vi "CUSUM_scan_histogram_20150428.vi"() -> ()   [LabVIEW 2012]
uses:
  <vilib>/Utility/file.llb/Read From Spreadsheet File (DBL).vi
  <vilib>/Analysis/NI_AALPro.lvlib
panel:
  out "Scatter density":i32[][](graph)
  in  "Log t":bool=TRUE
  in  "Min I (pA)":dbl format="%_3g"
  in  "Max I (pA)":dbl=1.0 format="%_3g"
  in  "Current bins":i16=100
  in  "t Min (us)":dbl=1.0 format="%_3g"
  in  "t Max (us)":dbl=2000000.0 format="%_3g"
  in  "t Bins":i16=100
  out "Blockage vs Event time":cluster{"all rows":dbl[], "all rows":dbl[]}(graph)={"all rows"=[1.5563025007672873, 2.041392685158225, 1.9444826721501687, 1.806179973983887, 2.0170333392987803, 1.7323937598229686, 2.1760912590556813, 2.2695129442179165, 2.662757831681574, 2.0644579892269186, 2.1760912590556813, 2.1072099696478683, 1.6434526764861874, 1.380211241711606, 2.2355284469075487, 2.4471580313422194, 1.954242509439325, 1.7481880270062005, 1.9030899869919435, 2.250420002308894, 1.4771212547196624, 2.606381365110605, 2.7781512503836434, 2.1760912590556813, 1.9637878273455553, 3.9774492273823414, 2.0086001717619175, 2.2600713879850747, 2.225309281725863, 2.113943352306837, 3.902655475217926, 1.4771212547196624, 3.45484486000851, 1.7160033436347992, 5.550074181736537, 2.1072099696478683, 2.100370545117563, 2.255272505103306, 2.093421685162235, 1.9242792860618816, 2.6020599913279625, 1.9912260756924949, 1.8325089127062364, 1.7481880270062005, 1.8920946026904804, 2.0, 1.8692317197309762, 1.6434526764861874, 1.9344984512435677, 3.5804687839510017, 2.0170333392987803, 1.792391689498254, 1.9138138523837167, 1.8573324964312685, 3.8290463368531826, 2.3909351071033793, 1.9138138523837167, 2.0569048513364727, 1.9344984512435677, 2.6085260335771943, 3.569373909615046, 2.230448921378274, 1.6812412373755872, 1.5314789170422551, 2.1583624920952498, 1.792391689498254, 1.6232492903979006, 1.9138138523837167, 1.8573324964312685, 1.9344984512435677, 1.7781512503836436, 1.9912260756924949, 1.9030899869919435, 3.1947917577219247, 1.5314789170422551, 1.9444826721501687, 2.230448921378274, 1.5314789170422551, 2.0791812460476247, 1.9822712330395684, 1.9444826721501687, 1.9138138523837167, 1.845098040014257, 1.5563025007672873, 1.9030899869919435, 1.9822712330395684, 2.4885507165004443, 1.6434526764861874, 3.9707187037201894, 1.6020599913279623, 1.7323937598229686, 1.8195439355418688, 1.8920946026904804, 1.6989700043360187, 2.1398790864012365, 2.4471580313422194, 1.414973347970818, 1.662757831681574, 1.9030899869919435, 4.0288151698468875, 4.322260654143684, 1.8692317197309762, 2.1335389083702174, 2.4771212547196626, 1.414973347970818, 3.396548037987132, 1.8325089127062364, 1.9242792860618816, 6.216878141702857], "all rows"=[0.0, 0.466725, 0.526039, 0.471183, 0.48709, 0.480192, 0.48409, 0.485169, 0.497506, 0.568502, 0.497117, 0.506935, 0.466185, 0.30941, 0.262762, 0.516642, 0.578892, 0.481172, 0.221123, 0.478859, 0.568097, 0.261814, 0.458444, 0.504733, 0.43433, 0.563135, 0.581725, 0.386148, 0.494293, 0.379628, 0.439002, 0.509173, 0.287608, 0.718087, 0.344776, 0.470972, 0.513751, 0.523004, 0.445567, 0.528748, 0.51793, 0.563512, 0.490711, 0.421606, 0.377698, 0.503034, 0.462329, 0.428095, 0.323342, 0.48743, 0.602688, 0.457485, 0.37527, 0.476058, 0.431685, 0.5739, 0.53304, 0.570076, 0.465926, 0.497023, 0.567974, 0.579427, 0.493678, 0.355429, 0.336341, 0.486281, 0.334836, 0.577798, 0.602408, 0.423267, 0.54713, 0.322654, 0.511843, 0.365353, 0.548216, 0.278652, 0.437687, 0.455942, 0.307252, 0.48448599999999997, 0.463501, 0.477843, 0.448573, 0.359273, 0.370335, 0.484589, 0.49994, 0.501483, 0.358317, 0.618115, 0.284756, 0.438673, 0.50125, 0.433369, 0.40958, 0.569745, 0.473801, 0.336148, 0.429861, 0.504048, 0.766676, 0.672518, 0.569512, 0.542499, 0.561967, 0.314494, 0.70292, 0.356469, 14.4165]}
  in  "Scatter plot":bool
  in  "stop 2":bool
  in  "stop":bool
  in  "Dwell time min bin":dbl format="%0.2f"
  in  "Dwell time max bin":dbl=20000.0 format="%0.2f"
  in  "Max block min (pA)":dbl format="%0.2f"
  in  "Max block max (pA)":dbl=1.0 format="%0.2f"
  in  "#bins (max block)":i32=50
  out "Max blockage (pA)":T1(graph)={"X Values"=[0.01, 0.03, 0.05, 0.07, 0.09, 0.11, 0.13, 0.15000000000000002, 0.16999999999999998, 0.19, 0.21000000000000002, 0.22999999999999998, 0.25, 0.27, 0.29000000000000004, 0.31, 0.33, 0.35, 0.37, 0.39, 0.41000000000000003, 0.43, 0.45, 0.47, 0.49, 0.51, 0.53, 0.55, 0.5700000000000001, 0.59, 0.61, 0.63, 0.65, 0.67, 0.6900000000000001, 0.71, 0.73, 0.75, 0.77, 0.79, 0.81, 0.8300000000000001, 0.85, 0.87, 0.89, 0.91, 0.93, 0.95, 0.97, 0.99], "Histogram: h(x)"=[0.0, 0.0, 0.0, 0.0, 0.0, 0.0, 0.0, 0.0, 0.0, 0.0, 0.0, 0.0, 0.0, 0.009345794392523364, 0.009345794392523364, 0.0, 0.018691588785046728, 0.018691588785046728, 0.06542056074766354, 0.009345794392523364, 0.056074766355140186, 0.028037383177570093, 0.06542056074766354, 0.07476635514018691, 0.09345794392523364, 0.14018691588785046, 0.14953271028037382, 0.037383177570093455, 0.08411214953271028, 0.06542056074766354, 0.018691588785046728, 0.009345794392523364, 0.0, 0.009345794392523364, 0.018691588785046728, 0.009345794392523364, 0.0, 0.0, 0.009345794392523364, 0.0, 0.0, 0.0, 0.0, 0.0, 0.0, 0.0, 0.0, 0.0, 0.0, 0.0]}
  out "Dwell time (us)":cluster{"Axis":dbl[], dbl[]}[](graph)=[{"Axis"=[200.0, 600.0, 1000.0, 1400.0, 1800.0, 2200.0, 2600.0, 3000.0, 3400.0, 3800.0, 4200.0, 4600.0, 5000.0, 5400.0, 5800.0, 6200.0, 6600.0, 7000.0, 7400.0, 7800.0, 8200.0, 8600.0, 9000.0, 9400.0, 9800.0, 10200.0, 10600.0, 11000.0, 11400.0, 11800.0, 12200.0, 12600.0, 13000.0, 13400.0, 13800.0, 14200.0, 14600.0, 15000.0, 15400.0, 15800.0, 16200.0, 16600.0, 17000.0, 17400.0, 17800.0, 18200.0, 18600.0, 19000.0, 19400.0, 19800.0], [91.0, 5.0, 0.0, 1.0, 0.0, 0.0, 1.0, 1.0, 0.0, 2.0, 0.0, 0.0, 0.0, 0.0, 0.0, 0.0, 1.0, 0.0, 0.0, 1.0, 0.0, 0.0, 0.0, 2.0, 0.0, 0.0, 1.0, 0.0, 0.0, 0.0, 0.0, 0.0, 0.0, 0.0, 0.0, 0.0, 0.0, 0.0, 0.0, 0.0, 0.0, 0.0, 0.0, 0.0, 0.0, 0.0, 0.0, 0.0, 0.0, 0.0]}, {"Axis"=[200.0, 600.0, 1000.0, 1400.0, 1800.0, 2200.0, 2600.0, 3000.0, 3400.0, 3800.0, 4200.0, 4600.0, 5000.0, 5400.0, 5800.0, 6200.0, 6600.0, 7000.0, 7400.0, 7800.0, 8200.0, 8600.0, 9000.0, 9400.0, 9800.0, 10200.0, 10600.0, 11000.0, 11400.0, 11800.0, 12200.0, 12600.0, 13000.0, 13400.0, 13800.0, 14200.0, 14600.0, 15000.0, 15400.0, 15800.0, 16200.0, 16600.0, 17000.0, 17400.0, 17800.0, 18200.0, 18600.0, 19000.0, 19400.0, 19800.0], [0.8584905660377359, 0.04716981132075472, 0.0, 0.009433962264150943, 0.0, 0.0, 0.009433962264150943, 0.009433962264150943, 0.0, 0.018867924528301886, 0.0, 0.0, 0.0, 0.0, 0.0, 0.0, 0.009433962264150943, 0.0, 0.0, 0.009433962264150943, 0.0, 0.0, 0.0, 0.018867924528301886, 0.0, 0.0, 0.009433962264150943, 0.0, 0.0, 0.0, 0.0, 0.0, 0.0, 0.0, 0.0, 0.0, 0.0, 0.0, 0.0, 0.0, 0.0, 0.0, 0.0, 0.0, 0.0, 0.0, 0.0, 0.0, 0.0, 0.0]}]
  out "min dwell time":dbl=24.0
  out "max dwell time":dbl=1647700.0
  in  "#bins (dwell)":i32=50
  in  "Max blockage histogram":bool
  in  "Dwell time histogram":bool
  out "Events analysed":i32
  out "sum (dummy check)":dbl=0.9807673664328832
  out "event length":i32=823856
  out "Histogram":i32[](array[numeric])
  out "Levels histogram":cluster{"Axis":dbl[], dbl[]}(graph)={"Axis"=[-2925.0, -2775.0, -2625.0, -2475.0, -2325.0, -2175.0, -2025.0, -1875.0, -1725.0, -1575.0, -1425.0, -1275.0, -1125.0, -975.0, -825.0, -675.0, -525.0, -375.0, -225.0, -75.0], [0.0, 0.0, 0.0, 0.0, 0.0, 0.0, 0.0, 0.0, 0.0, 0.0, 0.0, 0.00022756755787289165, 0.6987230927229675, 0.000277542494399701, 0.001647841378534532, 0.026337860039121676, 0.1949290617247068, 0.049781111930785465, 0.008843288584494536, 0.0]}
  out "Cumulative histogram":i32[](array[numeric])
  in  "# bins":i32=20
  in  "Min current (pA)":dbl=-3000.0 format="%0.2f"
  in  "Max current (pA)":dbl format="%0.2f"
  in  "CUSUM levels histogram":bool
  out "Event details":dbl[](array[numeric])=[12.97, 40.0, 729.134, 1.0] caption="Time (s)\n      Length (us)\nMax block (pA)   \n           # levels"
  out "CUSUM event":path=path "D:/Analysis/CUSUM_github/CUSUM/output/events/event_00000.csv"
  out "CUSUM event":cluster{"Y":dbl[], "Y":dbl[]}[](graph)=[{"Y"=[0.0, 2.0, 4.0, 6.0, 8.0, 10.0, 12.0, 14.0, 16.0, 18.0, 20.0, 22.0, 24.0, 26.0, 28.0, 30.0, 32.0, 34.0, 36.0, 38.0, 40.0, 42.0, 44.0, 46.0, 48.0, 50.0, 52.0, 54.0, 56.0, 58.0, 60.0, 62.0, 64.0, 66.0, 68.0, 70.0, 72.0, 74.0, 76.0, 78.0, 80.0, 82.0, 84.0, 86.0, 88.0, 90.0, 92.0, 94.0, 96.0, 98.0, 100.0, 102.0, 104.0, 106.0, 108.0, 110.0, 112.0, 114.0, 116.0, 118.0, 120.0, 122.0, 124.0, 126.0, 128.0, 130.0, 132.0, 134.0, 136.0, 138.0, 140.0, 142.0, 144.0, 146.0, 148.0, 150.0, 152.0, 154.0, 156.0, 158.0, 160.0, 162.0, 164.0, 166.0, 168.0, 170.0, 172.0, 174.0, 176.0, 178.0, 180.0, 182.0, 184.0, 186.0, 188.0, 190.0, 192.0, 194.0, 196.0, 198.0, 200.0, 202.0, 204.0, 206.0, 208.0, 210.0, 212.0, 214.0, 216.0, 218.0, 220.0, 222.0, 224.0, 226.0, 228.0, 230.0, 232.0, 234.0, 236.0, 238.0, 240.0, 242.0, 244.0, 246.0, 248.0, 250.0, 252.0, 254.0, 256.0, 258.0, 260.0, 262.0, 264.0, 266.0, 268.0, 270.0, 272.0, 274.0, 276.0, 278.0, 280.0, 282.0, 284.0, 286.0, 288.0, 290.0, 292.0, 294.0, 296.0, 298.0, 300.0, 302.0, 304.0, 306.0, 308.0, 310.0, 312.0, 314.0, 316.0, 318.0, 320.0, 322.0, 324.0, 326.0, 328.0, 330.0, 332.0, 334.0, 336.0, 338.0, 340.0, 342.0, 344.0, 346.0, 348.0, 350.0, 352.0, 354.0, 356.0, 358.0, 360.0, 362.0, 364.0, 366.0, 368.0, 370.0, 372.0, 374.0, 376.0, 378.0, 380.0, 382.0, 384.0, 386.0, 388.0, 390.0, 392.0, 394.0, 396.0, 398.0, 400.0, 402.0, 404.0, 406.0, 408.0, 410.0, 412.0, 414.0, 416.0, 418.0, 420.0, 422.0, 424.0, 426.0, 428.0, 430.0, 432.0, 434.0, 436.0, 438.0], "Y"=[-1508.27, -1508.27, -1508.27, -1508.27, -1508.27, -1508.27, -1508.27, -1508.27, -1508.27, -1508.27, -1508.27, -1508.27, -1508.27, -1508.27, -1508.27, -1508.27, -1508.27, -1508.27, -1508.27, -1508.27, -1508.27, -1508.27, -1508.27, -1508.27, -1508.27, -1508.27, -1508.27, -1508.27, -1508.27, -1508.27, -1508.27, -1508.27, -1508.27, -1508.27, -1508.27, -1508.27, -1508.27, -1508.27, -1508.27, -1508.27, -1508.27, -1508.27, -1508.27, -1508.27, -1508.27, -1508.27, -1508.27, -1508.27, -1508.27, -1508.27, -1508.27, -1508.27, -1508.27, -1508.27, -1508.27, -1508.27, -1508.27, -1508.27, -1508.27, -1508.27, -1508.27, -1508.27, -1508.27, -1508.27, -1508.27, -1508.27, -1508.27, -1508.27, -1508.27, -1508.27, -1508.27, -1508.27, -1508.27, -1508.27, -1508.27, -1508.27, -1508.27, -1508.27, -1508.27, -1508.27, -1508.27, -1508.27, -1508.27, -1508.27, -1508.27, -1508.27, -1508.27, -1508.27, -1508.27, -1508.27, -1508.27, -1508.27, -1508.27, -1508.27, -1508.27, -1508.27, -772.071, -772.071, -772.071, -772.071, -772.071, -772.071, -772.071, -772.071, -772.071, -772.071, -772.071, -772.071, -772.071, -772.071, -772.071, -772.071, -772.071, -772.071, -772.071, -772.071, -1508.61, -1508.61, -1508.61, -1508.61, -1508.61, -1508.61, -1508.61, -1508.61, -1508.61, -1508.61, -1508.61, -1508.61, -1508.61, -1508.61, -1508.61, -1508.61, -1508.61, -1508.61, -1508.61, -1508.61, -1508.61, -1508.61, -1508.61, -1508.61, -1508.61, -1508.61, -1508.61, -1508.61, -1508.61, -1508.61, -1508.61, -1508.61, -1508.61, -1508.61, -1508.61, -1508.61, -1508.61, -1508.61, -1508.61, -1508.61, -1508.61, -1508.61, -1508.61, -1508.61, -1508.61, -1508.61, -1508.61, -1508.61, -1508.61, -1508.61, -1508.61, -1508.61, -1508.61, -1508.61, -1508.61, -1508.61, -1508.61, -1508.61, -1508.61, -1508.61, -1508.61, -1508.61, -1508.61, -1508.61, -1508.61, -1508.61, -1508.61, -1508.61, -1508.61, -1508.61, -1508.61, -1508.61, -1508.61, -1508.61, -1508.61, -1508.61, -1508.61, -1508.61, -1508.61, -1508.61, -1508.61, -1508.61, -1508.61, -1508.61, -1508.61, -1508.61, -1508.61, -1508.61, -1508.61, -1508.61, -1508.61, -1508.61, -1508.61, -1508.61, -1508.61, -1508.61, -1508.61, -1508.61, -1508.61, -1508.61, -1508.61, -1508.61, -1508.61, -1508.61]}, {"Y"=[0.0, 2.0, 4.0, 6.0, 8.0, 10.0, 12.0, 14.0, 16.0, 18.0, 20.0, 22.0, 24.0, 26.0, 28.0, 30.0, 32.0, 34.0, 36.0, 38.0, 40.0, 42.0, 44.0, 46.0, 48.0, 50.0, 52.0, 54.0, 56.0, 58.0, 60.0, 62.0, 64.0, 66.0, 68.0, 70.0, 72.0, 74.0, 76.0, 78.0, 80.0, 82.0, 84.0, 86.0, 88.0, 90.0, 92.0, 94.0, 96.0, 98.0, 100.0, 102.0, 104.0, 106.0, 108.0, 110.0, 112.0, 114.0, 116.0, 118.0, 120.0, 122.0, 124.0, 126.0, 128.0, 130.0, 132.0, 134.0, 136.0, 138.0, 140.0, 142.0, 144.0, 146.0, 148.0, 150.0, 152.0, 154.0, 156.0, 158.0, 160.0, 162.0, 164.0, 166.0, 168.0, 170.0, 172.0, 174.0, 176.0, 178.0, 180.0, 182.0, 184.0, 186.0, 188.0, 190.0, 192.0, 194.0, 196.0, 198.0, 200.0, 202.0, 204.0, 206.0, 208.0, 210.0, 212.0, 214.0, 216.0, 218.0, 220.0, 222.0, 224.0, 226.0, 228.0, 230.0, 232.0, 234.0, 236.0, 238.0, 240.0, 242.0, 244.0, 246.0, 248.0, 250.0, 252.0, 254.0, 256.0, 258.0, 260.0, 262.0, 264.0, 266.0, 268.0, 270.0, 272.0, 274.0, 276.0, 278.0, 280.0, 282.0, 284.0, 286.0, 288.0, 290.0, 292.0, 294.0, 296.0, 298.0, 300.0, 302.0, 304.0, 306.0, 308.0, 310.0, 312.0, 314.0, 316.0, 318.0, 320.0, 322.0, 324.0, 326.0, 328.0, 330.0, 332.0, 334.0, 336.0, 338.0, 340.0, 342.0, 344.0, 346.0, 348.0, 350.0, 352.0, 354.0, 356.0, 358.0, 360.0, 362.0, 364.0, 366.0, 368.0, 370.0, 372.0, 374.0, 376.0, 378.0, 380.0, 382.0, 384.0, 386.0, 388.0, 390.0, 392.0, 394.0, 396.0, 398.0, 400.0, 402.0, 404.0, 406.0, 408.0, 410.0, 412.0, 414.0, 416.0, 418.0, 420.0, 422.0, 424.0, 426.0, 428.0, 430.0, 432.0, 434.0, 436.0, 438.0], "Y"=[-1591.0, -1421.0, -1377.0, -1507.0, -1587.0, -1555.0, -1525.0, -1599.0, -1675.0, -1611.0, -1522.0, -1485.0, -1503.0, -1599.0, -1521.0, -1314.0, -1273.0, -1460.0, -1603.0, -1536.0, -1415.0, -1464.0, -1619.0, -1713.0, -1672.0, -1504.0, -1475.0, -1558.0, -1529.0, -1446.0, -1411.0, -1400.0, -1501.0, -1613.0, -1571.0, -1472.0, -1484.0, -1538.0, -1437.0, -1313.0, -1363.0, -1463.0, -1461.0, -1390.0, -1323.0, -1322.0, -1513.0, -1657.0, -1618.0, -1466.0, -1355.0, -1465.0, -1560.0, -1517.0, -1441.0, -1459.0, -1398.0, -1396.0, -1455.0, -1489.0, -1574.0, -1630.0, -1561.0, -1525.0, -1483.0, -1555.0, -1600.0, -1542.0, -1463.0, -1484.0, -1550.0, -1559.0, -1489.0, -1380.0, -1454.0, -1640.0, -1731.0, -1722.0, -1512.0, -1454.0, -1525.0, -1579.0, -1514.0, -1447.0, -1563.0, -1594.0, -1434.0, -1364.0, -1457.0, -1674.0, -1679.0, -1552.0, -1467.0, -1450.0, -1532.0, -1533.0, -1326.0, -1135.0, -1060.0, -1000.0, -855.0, -654.0, -599.0, -706.0, -794.0, -828.0, -804.0, -746.0, -802.0, -892.0, -790.0, -635.0, -657.0, -792.0, -907.0, -857.0, -924.0, -1202.0, -1410.0, -1325.0, -1275.0, -1315.0, -1432.0, -1525.0, -1512.0, -1491.0, -1390.0, -1342.0, -1478.0, -1581.0, -1497.0, -1437.0, -1585.0, -1622.0, -1547.0, -1561.0, -1547.0, -1516.0, -1443.0, -1399.0, -1358.0, -1423.0, -1571.0, -1589.0, -1513.0, -1480.0, -1594.0, -1705.0, -1670.0, -1530.0, -1461.0, -1530.0, -1554.0, -1438.0, -1399.0, -1421.0, -1506.0, -1549.0, -1498.0, -1375.0, -1339.0, -1460.0, -1545.0, -1444.0, -1327.0, -1458.0, -1582.0, -1587.0, -1582.0, -1545.0, -1614.0, -1637.0, -1503.0, -1391.0, -1356.0, -1405.0, -1457.0, -1506.0, -1503.0, -1450.0, -1527.0, -1602.0, -1546.0, -1399.0, -1443.0, -1593.0, -1650.0, -1594.0, -1517.0, -1546.0, -1696.0, -1683.0, -1579.0, -1548.0, -1611.0, -1620.0, -1542.0, -1484.0, -1450.0, -1508.0, -1537.0, -1490.0, -1448.0, -1432.0, -1527.0, -1578.0, -1494.0, -1408.0, -1424.0, -1537.0, -1626.0, -1617.0, -1508.0, -1456.0, -1497.0, -1514.0, -1427.0, -1400.0, -1502.0, -1599.0]}]
  in  "Event Index":i32
  out "All Files in Dir":path[](array[path])=[path "D:/Analysis/CUSUM_github/CUSUM/output/events/event_00000.csv", path "D:/Analysis/CUSUM_github/CUSUM/output/events/event_00001.csv", path "D:/Analysis/CUSUM_github/CUSUM/output/events/event_00004.csv", path "D:/Analysis/CUSUM_github/CUSUM/output/events/event_00009.csv", path "D:/Analysis/CUSUM_github/CUSUM/output/events/event_00011.csv", path "D:/Analysis/CUSUM_github/CUSUM/output/events/event_00013.csv", path "D:/Analysis/CUSUM_github/CUSUM/output/events/event_00015.csv", path "D:/Analysis/CUSUM_github/CUSUM/output/events/event_00016.csv", path "D:/Analysis/CUSUM_github/CUSUM/output/events/event_00018.csv", path "D:/Analysis/CUSUM_github/CUSUM/output/events/event_00019.csv", path "D:/Analysis/CUSUM_github/CUSUM/output/events/event_00020.csv", path "D:/Analysis/CUSUM_github/CUSUM/output/events/event_00022.csv", path "D:/Analysis/CUSUM_github/CUSUM/output/events/event_00024.csv", path "D:/Analysis/CUSUM_github/CUSUM/output/events/event_00025.csv", path "D:/Analysis/CUSUM_github/CUSUM/output/events/event_00027.csv", path "D:/Analysis/CUSUM_github/CUSUM/output/events/event_00031.csv", path "D:/Analysis/CUSUM_github/CUSUM/output/events/event_00032.csv", path "D:/Analysis/CUSUM_github/CUSUM/output/events/event_00034.csv", path "D:/Analysis/CUSUM_github/CUSUM/output/events/event_00035.csv", path "D:/Analysis/CUSUM_github/CUSUM/output/events/event_00038.csv", path "D:/Analysis/CUSUM_github/CUSUM/output/events/event_00041.csv", path "D:/Analysis/CUSUM_github/CUSUM/output/events/event_00043.csv", path "D:/Analysis/CUSUM_github/CUSUM/output/events/event_00044.csv", path "D:/Analysis/CUSUM_github/CUSUM/output/events/event_00046.csv", path "D:/Analysis/CUSUM_github/CUSUM/output/events/event_00047.csv", path "D:/Analysis/CUSUM_github/CUSUM/output/events/event_00048.csv", path "D:/Analysis/CUSUM_github/CUSUM/output/events/event_00049.csv", path "D:/Analysis/CUSUM_github/CUSUM/output/events/event_00051.csv", path "D:/Analysis/CUSUM_github/CUSUM/output/events/event_00053.csv", path "D:/Analysis/CUSUM_github/CUSUM/output/events/event_00054.csv", path "D:/Analysis/CUSUM_github/CUSUM/output/events/event_00056.csv", path "D:/Analysis/CUSUM_github/CUSUM/output/events/event_00057.csv", path "D:/Analysis/CUSUM_github/CUSUM/output/events/event_00060.csv", path "D:/Analysis/CUSUM_github/CUSUM/output/events/event_00061.csv", path "D:/Analysis/CUSUM_github/CUSUM/output/events/event_00062.csv", path "D:/Analysis/CUSUM_github/CUSUM/output/events/event_00063.csv", path "D:/Analysis/CUSUM_github/CUSUM/output/events/event_00068.csv", path "D:/Analysis/CUSUM_github/CUSUM/output/events/event_00069.csv", path "D:/Analysis/CUSUM_github/CUSUM/output/events/event_00070.csv", path "D:/Analysis/CUSUM_github/CUSUM/output/events/event_00072.csv", path "D:/Analysis/CUSUM_github/CUSUM/output/events/event_00074.csv", path "D:/Analysis/CUSUM_github/CUSUM/output/events/event_00076.csv", path "D:/Analysis/CUSUM_github/CUSUM/output/events/event_00077.csv", path "D:/Analysis/CUSUM_github/CUSUM/output/events/event_00078.csv", path "D:/Analysis/CUSUM_github/CUSUM/output/events/event_00079.csv", path "D:/Analysis/CUSUM_github/CUSUM/output/events/event_00080.csv", path "D:/Analysis/CUSUM_github/CUSUM/output/events/event_00081.csv", path "D:/Analysis/CUSUM_github/CUSUM/output/events/event_00082.csv", path "D:/Analysis/CUSUM_github/CUSUM/output/events/event_00084.csv", path "D:/Analysis/CUSUM_github/CUSUM/output/events/event_00087.csv", path "D:/Analysis/CUSUM_github/CUSUM/output/events/event_00089.csv", path "D:/Analysis/CUSUM_github/CUSUM/output/events/event_00093.csv", path "D:/Analysis/CUSUM_github/CUSUM/output/events/event_00094.csv", path "D:/Analysis/CUSUM_github/CUSUM/output/events/event_00096.csv", path "D:/Analysis/CUSUM_github/CUSUM/output/events/event_00098.csv", path "D:/Analysis/CUSUM_github/CUSUM/output/events/event_00101.csv", path "D:/Analysis/CUSUM_github/CUSUM/output/events/event_00102.csv", path "D:/Analysis/CUSUM_github/CUSUM/output/events/event_00103.csv", path "D:/Analysis/CUSUM_github/CUSUM/output/events/event_00108.csv", path "D:/Analysis/CUSUM_github/CUSUM/output/events/event_00109.csv", path "D:/Analysis/CUSUM_github/CUSUM/output/events/event_00111.csv", path "D:/Analysis/CUSUM_github/CUSUM/output/events/event_00114.csv", path "D:/Analysis/CUSUM_github/CUSUM/output/events/event_00120.csv", path "D:/Analysis/CUSUM_github/CUSUM/output/events/event_00121.csv", path "D:/Analysis/CUSUM_github/CUSUM/output/events/event_00122.csv", path "D:/Analysis/CUSUM_github/CUSUM/output/events/event_00128.csv", path "D:/Analysis/CUSUM_github/CUSUM/output/events/event_00130.csv", path "D:/Analysis/CUSUM_github/CUSUM/output/events/event_00131.csv", path "D:/Analysis/CUSUM_github/CUSUM/output/events/event_00132.csv", path "D:/Analysis/CUSUM_github/CUSUM/output/events/event_00133.csv", path "D:/Analysis/CUSUM_github/CUSUM/output/events/event_00134.csv", path "D:/Analysis/CUSUM_github/CUSUM/output/events/event_00137.csv", path "D:/Analysis/CUSUM_github/CUSUM/output/events/event_00138.csv", path "D:/Analysis/CUSUM_github/CUSUM/output/events/event_00139.csv", path "D:/Analysis/CUSUM_github/CUSUM/output/events/event_00142.csv", path "D:/Analysis/CUSUM_github/CUSUM/output/events/event_00143.csv", path "D:/Analysis/CUSUM_github/CUSUM/output/events/event_00146.csv", path "D:/Analysis/CUSUM_github/CUSUM/output/events/event_00148.csv", path "D:/Analysis/CUSUM_github/CUSUM/output/events/event_00152.csv", path "D:/Analysis/CUSUM_github/CUSUM/output/events/event_00155.csv", path "D:/Analysis/CUSUM_github/CUSUM/output/events/event_00156.csv", path "D:/Analysis/CUSUM_github/CUSUM/output/events/event_00164.csv", path "D:/Analysis/CUSUM_github/CUSUM/output/events/event_00166.csv", path "D:/Analysis/CUSUM_github/CUSUM/output/events/event_00167.csv", path "D:/Analysis/CUSUM_github/CUSUM/output/events/event_00171.csv", path "D:/Analysis/CUSUM_github/CUSUM/output/events/event_00172.csv", path "D:/Analysis/CUSUM_github/CUSUM/output/events/event_00176.csv", path "D:/Analysis/CUSUM_github/CUSUM/output/events/event_00177.csv", path "D:/Analysis/CUSUM_github/CUSUM/output/events/event_00178.csv", path "D:/Analysis/CUSUM_github/CUSUM/output/events/event_00181.csv", path "D:/Analysis/CUSUM_github/CUSUM/output/events/event_00187.csv", path "D:/Analysis/CUSUM_github/CUSUM/output/events/event_00189.csv", path "D:/Analysis/CUSUM_github/CUSUM/output/events/event_00193.csv", path "D:/Analysis/CUSUM_github/CUSUM/output/events/event_00195.csv", path "D:/Analysis/CUSUM_github/CUSUM/output/events/event_00196.csv", path "D:/Analysis/CUSUM_github/CUSUM/output/events/event_00197.csv", path "D:/Analysis/CUSUM_github/CUSUM/output/events/event_00203.csv", path "D:/Analysis/CUSUM_github/CUSUM/output/events/event_00204.csv", path "D:/Analysis/CUSUM_github/CUSUM/output/events/event_00205.csv", path "D:/Analysis/CUSUM_github/CUSUM/output/events/event_00208.csv", path "D:/Analysis/CUSUM_github/CUSUM/output/events/event_00209.csv", path "D:/Analysis/CUSUM_github/CUSUM/output/events/event_00210.csv", path "D:/Analysis/CUSUM_github/CUSUM/output/events/event_00211.csv", path "D:/Analysis/CUSUM_github/CUSUM/output/events/event_00212.csv", path "D:/Analysis/CUSUM_github/CUSUM/output/events/event_00213.csv", path "D:/Analysis/CUSUM_github/CUSUM/output/events/event_00216.csv", path "D:/Analysis/CUSUM_github/CUSUM/output/events/event_00218.csv", path "D:/Analysis/CUSUM_github/CUSUM/output/events/event_00221.csv", path "D:/Analysis/CUSUM_github/CUSUM/output/events/event_00222.csv", path "D:/Analysis/CUSUM_github/CUSUM/output/events/event_00223.csv", path "D:/Analysis/CUSUM_github/CUSUM/output/events/event_00230.csv", path "D:/Analysis/CUSUM_github/CUSUM/output/events/event_00232.csv", path "D:/Analysis/CUSUM_github/CUSUM/output/events/event_00233.csv", path "D:/Analysis/CUSUM_github/CUSUM/output/events/event_00234.csv", path "D:/Analysis/CUSUM_github/CUSUM/output/events/event_00238.csv", path "D:/Analysis/CUSUM_github/CUSUM/output/events/event_00240.csv", path "D:/Analysis/CUSUM_github/CUSUM/output/events/event_00247.csv", path "D:/Analysis/CUSUM_github/CUSUM/output/events/event_00249.csv", path "D:/Analysis/CUSUM_github/CUSUM/output/events/event_00255.csv", path "D:/Analysis/CUSUM_github/CUSUM/output/events/event_00257.csv", path "D:/Analysis/CUSUM_github/CUSUM/output/events/event_00258.csv", path "D:/Analysis/CUSUM_github/CUSUM/output/events/event_00264.csv", path "D:/Analysis/CUSUM_github/CUSUM/output/events/event_00265.csv", path "D:/Analysis/CUSUM_github/CUSUM/output/events/event_00267.csv", path "D:/Analysis/CUSUM_github/CUSUM/output/events/event_00268.csv", path "D:/Analysis/CUSUM_github/CUSUM/output/events/event_00271.csv", path "D:/Analysis/CUSUM_github/CUSUM/output/events/event_00273.csv", path "D:/Analysis/CUSUM_github/CUSUM/output/events/event_00280.csv", path "D:/Analysis/CUSUM_github/CUSUM/output/events/event_00285.csv", path "D:/Analysis/CUSUM_github/CUSUM/output/events/event_00286.csv", path "D:/Analysis/CUSUM_github/CUSUM/output/events/event_00287.csv", path "D:/Analysis/CUSUM_github/CUSUM/output/events/event_00288.csv", path "D:/Analysis/CUSUM_github/CUSUM/output/events/event_00289.csv", path "D:/Analysis/CUSUM_github/CUSUM/output/events/event_00290.csv", path "D:/Analysis/CUSUM_github/CUSUM/output/events/event_00291.csv", path "D:/Analysis/CUSUM_github/CUSUM/output/events/event_00294.csv", path "D:/Analysis/CUSUM_github/CUSUM/output/events/event_00297.csv", path "D:/Analysis/CUSUM_github/CUSUM/output/events/event_00300.csv", path "D:/Analysis/CUSUM_github/CUSUM/output/events/event_00302.csv", path "D:/Analysis/CUSUM_github/CUSUM/output/events/event_00305.csv", path "D:/Analysis/CUSUM_github/CUSUM/output/events/event_00306.csv", path "D:/Analysis/CUSUM_github/CUSUM/output/events/event_00307.csv", path "D:/Analysis/CUSUM_github/CUSUM/output/events/event_00308.csv", path "D:/Analysis/CUSUM_github/CUSUM/output/events/event_00310.csv", path "D:/Analysis/CUSUM_github/CUSUM/output/events/event_00313.csv", path "D:/Analysis/CUSUM_github/CUSUM/output/events/event_00317.csv", path "D:/Analysis/CUSUM_github/CUSUM/output/events/event_00319.csv", path "D:/Analysis/CUSUM_github/CUSUM/output/events/event_00322.csv", path "D:/Analysis/CUSUM_github/CUSUM/output/events/event_00323.csv", path "D:/Analysis/CUSUM_github/CUSUM/output/events/event_00324.csv", path "D:/Analysis/CUSUM_github/CUSUM/output/events/event_00325.csv", path "D:/Analysis/CUSUM_github/CUSUM/output/events/event_00328.csv", path "D:/Analysis/CUSUM_github/CUSUM/output/events/event_00331.csv", path "D:/Analysis/CUSUM_github/CUSUM/output/events/event_00332.csv", path "D:/Analysis/CUSUM_github/CUSUM/output/events/event_00333.csv", path "D:/Analysis/CUSUM_github/CUSUM/output/events/event_00335.csv", path "D:/Analysis/CUSUM_github/CUSUM/output/events/event_00336.csv", path "D:/Analysis/CUSUM_github/CUSUM/output/events/event_00337.csv", path "D:/Analysis/CUSUM_github/CUSUM/output/events/event_00339.csv", path "D:/Analysis/CUSUM_github/CUSUM/output/events/event_00344.csv", path "D:/Analysis/CUSUM_github/CUSUM/output/events/event_00345.csv", path "D:/Analysis/CUSUM_github/CUSUM/output/events/event_00351.csv", path "D:/Analysis/CUSUM_github/CUSUM/output/events/event_00352.csv", path "D:/Analysis/CUSUM_github/CUSUM/output/events/event_00354.csv", path "D:/Analysis/CUSUM_github/CUSUM/output/events/event_00355.csv", path "D:/Analysis/CUSUM_github/CUSUM/output/events/event_00356.csv", path "D:/Analysis/CUSUM_github/CUSUM/output/events/event_00361.csv", path "D:/Analysis/CUSUM_github/CUSUM/output/events/event_00362.csv", path "D:/Analysis/CUSUM_github/CUSUM/output/events/event_00365.csv", path "D:/Analysis/CUSUM_github/CUSUM/output/events/event_00367.csv", path "D:/Analysis/CUSUM_github/CUSUM/output/events/event_00369.csv", path "D:/Analysis/CUSUM_github/CUSUM/output/events/event_00373.csv", path "D:/Analysis/CUSUM_github/CUSUM/output/events/event_00374.csv", path "D:/Analysis/CUSUM_github/CUSUM/output/events/event_00376.csv", path "D:/Analysis/CUSUM_github/CUSUM/output/events/event_00377.csv", path "D:/Analysis/CUSUM_github/CUSUM/output/events/event_00378.csv", path "D:/Analysis/CUSUM_github/CUSUM/output/events/event_00380.csv", path "D:/Analysis/CUSUM_github/CUSUM/output/events/event_00381.csv", path "D:/Analysis/CUSUM_github/CUSUM/output/events/event_00387.csv", path "D:/Analysis/CUSUM_github/CUSUM/output/events/event_00388.csv", path "D:/Analysis/CUSUM_github/CUSUM/output/events/event_00389.csv", path "D:/Analysis/CUSUM_github/CUSUM/output/events/event_00390.csv", path "D:/Analysis/CUSUM_github/CUSUM/output/events/event_00391.csv", path "D:/Analysis/CUSUM_github/CUSUM/output/events/event_00397.csv", path "D:/Analysis/CUSUM_github/CUSUM/output/events/event_00398.csv", path "D:/Analysis/CUSUM_github/CUSUM/output/events/event_00399.csv", path "D:/Analysis/CUSUM_github/CUSUM/output/events/event_00400.csv", path "D:/Analysis/CUSUM_github/CUSUM/output/events/event_00402.csv", path "D:/Analysis/CUSUM_github/CUSUM/output/events/event_00403.csv", path "D:/Analysis/CUSUM_github/CUSUM/output/events/event_00404.csv", path "D:/Analysis/CUSUM_github/CUSUM/output/events/event_00409.csv", path "D:/Analysis/CUSUM_github/CUSUM/output/events/event_00410.csv", path "D:/Analysis/CUSUM_github/CUSUM/output/events/event_00414.csv", path "D:/Analysis/CUSUM_github/CUSUM/output/events/event_00417.csv", path "D:/Analysis/CUSUM_github/CUSUM/output/events/event_00418.csv", path "D:/Analysis/CUSUM_github/CUSUM/output/events/event_00421.csv", path "D:/Analysis/CUSUM_github/CUSUM/output/events/event_00425.csv", path "D:/Analysis/CUSUM_github/CUSUM/output/events/event_00426.csv", path "D:/Analysis/CUSUM_github/CUSUM/output/events/event_00432.csv", path "D:/Analysis/CUSUM_github/CUSUM/output/events/event_00433.csv", path "D:/Analysis/CUSUM_github/CUSUM/output/events/event_00434.csv", path "D:/Analysis/CUSUM_github/CUSUM/output/events/event_00436.csv", path "D:/Analysis/CUSUM_github/CUSUM/output/events/event_00437.csv", path "D:/Analysis/CUSUM_github/CUSUM/output/events/event_00440.csv", path "D:/Analysis/CUSUM_github/CUSUM/output/events/event_00441.csv", path "D:/Analysis/CUSUM_github/CUSUM/output/events/event_00447.csv", path "D:/Analysis/CUSUM_github/CUSUM/output/events/event_00452.csv", path "D:/Analysis/CUSUM_github/CUSUM/output/events/event_00455.csv", path "D:/Analysis/CUSUM_github/CUSUM/output/events/event_00460.csv", path "D:/Analysis/CUSUM_github/CUSUM/output/events/event_00461.csv", path "D:/Analysis/CUSUM_github/CUSUM/output/events/event_00464.csv", path "D:/Analysis/CUSUM_github/CUSUM/output/events/event_00466.csv", path "D:/Analysis/CUSUM_github/CUSUM/output/events/event_00467.csv", path "D:/Analysis/CUSUM_github/CUSUM/output/events/event_00469.csv", path "D:/Analysis/CUSUM_github/CUSUM/output/events/event_00471.csv", path "D:/Analysis/CUSUM_github/CUSUM/output/events/event_00472.csv", path "D:/Analysis/CUSUM_github/CUSUM/output/events/event_00473.csv", path "D:/Analysis/CUSUM_github/CUSUM/output/events/event_00474.csv", path "D:/Analysis/CUSUM_github/CUSUM/output/events/event_00476.csv", path "D:/Analysis/CUSUM_github/CUSUM/output/events/event_00477.csv", path "D:/Analysis/CUSUM_github/CUSUM/output/events/event_00478.csv", path "D:/Analysis/CUSUM_github/CUSUM/output/events/event_00480.csv", path "D:/Analysis/CUSUM_github/CUSUM/output/events/event_00484.csv", path "D:/Analysis/CUSUM_github/CUSUM/output/events/event_00485.csv", path "D:/Analysis/CUSUM_github/CUSUM/output/events/event_00487.csv", path "D:/Analysis/CUSUM_github/CUSUM/output/events/event_00488.csv", path "D:/Analysis/CUSUM_github/CUSUM/output/events/event_00490.csv", path "D:/Analysis/CUSUM_github/CUSUM/output/events/event_00495.csv", path "D:/Analysis/CUSUM_github/CUSUM/output/events/event_00501.csv", path "D:/Analysis/CUSUM_github/CUSUM/output/events/event_00504.csv", path "D:/Analysis/CUSUM_github/CUSUM/output/events/event_00506.csv", path "D:/Analysis/CUSUM_github/CUSUM/output/events/event_00507.csv", path "D:/Analysis/CUSUM_github/CUSUM/output/events/event_00508.csv", path "D:/Analysis/CUSUM_github/CUSUM/output/events/event_00509.csv", path "D:/Analysis/CUSUM_github/CUSUM/output/events/event_00510.csv", path "D:/Analysis/CUSUM_github/CUSUM/output/events/event_00512.csv", path "D:/Analysis/CUSUM_github/CUSUM/output/events/event_00515.csv", path "D:/Analysis/CUSUM_github/CUSUM/output/events/event_00516.csv", path "D:/Analysis/CUSUM_github/CUSUM/output/events/event_00517.csv", path "D:/Analysis/CUSUM_github/CUSUM/output/events/event_00525.csv", path "D:/Analysis/CUSUM_github/CUSUM/output/events/event_00526.csv", path "D:/Analysis/CUSUM_github/CUSUM/output/events/event_00527.csv", path "D:/Analysis/CUSUM_github/CUSUM/output/events/event_00531.csv", path "D:/Analysis/CUSUM_github/CUSUM/output/events/event_00533.csv", path "D:/Analysis/CUSUM_github/CUSUM/output/events/event_00534.csv", path "D:/Analysis/CUSUM_github/CUSUM/output/events/event_00535.csv", path "D:/Analysis/CUSUM_github/CUSUM/output/events/event_00539.csv", path "D:/Analysis/CUSUM_github/CUSUM/output/events/event_00540.csv", path "D:/Analysis/CUSUM_github/CUSUM/output/events/event_00544.csv", path "D:/Analysis/CUSUM_github/CUSUM/output/events/event_00547.csv", path "D:/Analysis/CUSUM_github/CUSUM/output/events/event_00548.csv", path "D:/Analysis/CUSUM_github/CUSUM/output/events/event_00551.csv", path "D:/Analysis/CUSUM_github/CUSUM/output/events/event_00553.csv", path "D:/Analysis/CUSUM_github/CUSUM/output/events/event_00556.csv", path "D:/Analysis/CUSUM_github/CUSUM/output/events/event_00557.csv", path "D:/Analysis/CUSUM_github/CUSUM/output/events/event_00558.csv", path "D:/Analysis/CUSUM_github/CUSUM/output/events/event_00561.csv", path "D:/Analysis/CUSUM_github/CUSUM/output/events/event_00563.csv", path "D:/Analysis/CUSUM_github/CUSUM/output/events/event_00564.csv", path "D:/Analysis/CUSUM_github/CUSUM/output/events/event_00566.csv", path "D:/Analysis/CUSUM_github/CUSUM/output/events/event_00567.csv", path "D:/Analysis/CUSUM_github/CUSUM/output/events/event_00568.csv", path "D:/Analysis/CUSUM_github/CUSUM/output/events/event_00569.csv", path "D:/Analysis/CUSUM_github/CUSUM/output/events/event_00570.csv", path "D:/Analysis/CUSUM_github/CUSUM/output/events/event_00576.csv", path "D:/Analysis/CUSUM_github/CUSUM/output/events/event_00577.csv", path "D:/Analysis/CUSUM_github/CUSUM/output/events/event_00580.csv", path "D:/Analysis/CUSUM_github/CUSUM/output/events/event_00585.csv", path "D:/Analysis/CUSUM_github/CUSUM/output/events/event_00586.csv", path "D:/Analysis/CUSUM_github/CUSUM/output/events/event_00589.csv", path "D:/Analysis/CUSUM_github/CUSUM/output/events/event_00592.csv", path "D:/Analysis/CUSUM_github/CUSUM/output/events/event_00595.csv", path "D:/Analysis/CUSUM_github/CUSUM/output/events/event_00597.csv", path "D:/Analysis/CUSUM_github/CUSUM/output/events/event_00598.csv", path "D:/Analysis/CUSUM_github/CUSUM/output/events/event_00599.csv", path "D:/Analysis/CUSUM_github/CUSUM/output/events/event_00606.csv", path "D:/Analysis/CUSUM_github/CUSUM/output/events/event_00608.csv", path "D:/Analysis/CUSUM_github/CUSUM/output/events/event_00609.csv", path "D:/Analysis/CUSUM_github/CUSUM/output/events/event_00610.csv", path "D:/Analysis/CUSUM_github/CUSUM/output/events/event_00611.csv", path "D:/Analysis/CUSUM_github/CUSUM/output/events/event_00614.csv", path "D:/Analysis/CUSUM_github/CUSUM/output/events/event_00615.csv", path "D:/Analysis/CUSUM_github/CUSUM/output/events/event_00616.csv", path "D:/Analysis/CUSUM_github/CUSUM/output/events/event_00617.csv", path "D:/Analysis/CUSUM_github/CUSUM/output/events/event_00618.csv", path "D:/Analysis/CUSUM_github/CUSUM/output/events/event_00624.csv", path "D:/Analysis/CUSUM_github/CUSUM/output/events/event_00625.csv", path "D:/Analysis/CUSUM_github/CUSUM/output/events/event_00626.csv", path "D:/Analysis/CUSUM_github/CUSUM/output/events/event_00628.csv", path "D:/Analysis/CUSUM_github/CUSUM/output/events/event_00630.csv", path "D:/Analysis/CUSUM_github/CUSUM/output/events/event_00632.csv", path "D:/Analysis/CUSUM_github/CUSUM/output/events/event_00633.csv", path "D:/Analysis/CUSUM_github/CUSUM/output/events/event_00634.csv", path "D:/Analysis/CUSUM_github/CUSUM/output/events/event_00635.csv", path "D:/Analysis/CUSUM_github/CUSUM/output/events/event_00636.csv", path "D:/Analysis/CUSUM_github/CUSUM/output/events/event_00638.csv", path "D:/Analysis/CUSUM_github/CUSUM/output/events/event_00640.csv", path "D:/Analysis/CUSUM_github/CUSUM/output/events/event_00649.csv", path "D:/Analysis/CUSUM_github/CUSUM/output/events/event_00655.csv", path "D:/Analysis/CUSUM_github/CUSUM/output/events/event_00659.csv", path "D:/Analysis/CUSUM_github/CUSUM/output/events/event_00666.csv", path "D:/Analysis/CUSUM_github/CUSUM/output/events/event_00669.csv", path "D:/Analysis/CUSUM_github/CUSUM/output/events/event_00670.csv", path "D:/Analysis/CUSUM_github/CUSUM/output/events/event_00673.csv", path "D:/Analysis/CUSUM_github/CUSUM/output/events/event_00679.csv", path "D:/Analysis/CUSUM_github/CUSUM/output/events/event_00694.csv", path "D:/Analysis/CUSUM_github/CUSUM/output/events/event_00698.csv", path "D:/Analysis/CUSUM_github/CUSUM/output/events/event_00700.csv", path "D:/Analysis/CUSUM_github/CUSUM/output/events/event_00701.csv", path "D:/Analysis/CUSUM_github/CUSUM/output/events/event_00702.csv", path "D:/Analysis/CUSUM_github/CUSUM/output/events/event_00703.csv", path "D:/Analysis/CUSUM_github/CUSUM/output/events/event_00707.csv", path "D:/Analysis/CUSUM_github/CUSUM/output/events/event_00708.csv", path "D:/Analysis/CUSUM_github/CUSUM/output/events/event_00709.csv", path "D:/Analysis/CUSUM_github/CUSUM/output/events/event_00710.csv", path "D:/Analysis/CUSUM_github/CUSUM/output/events/event_00713.csv", path "D:/Analysis/CUSUM_github/CUSUM/output/events/event_00716.csv", path "D:/Analysis/CUSUM_github/CUSUM/output/events/event_00717.csv", path "D:/Analysis/CUSUM_github/CUSUM/output/events/event_00718.csv", path "D:/Analysis/CUSUM_github/CUSUM/output/events/event_00720.csv", path "D:/Analysis/CUSUM_github/CUSUM/output/events/event_00721.csv", path "D:/Analysis/CUSUM_github/CUSUM/output/events/event_00723.csv", path "D:/Analysis/CUSUM_github/CUSUM/output/events/event_00724.csv", path "D:/Analysis/CUSUM_github/CUSUM/output/events/event_00726.csv", path "D:/Analysis/CUSUM_github/CUSUM/output/events/event_00728.csv", path "D:/Analysis/CUSUM_github/CUSUM/output/events/event_00731.csv", path "D:/Analysis/CUSUM_github/CUSUM/output/events/event_00732.csv", path "D:/Analysis/CUSUM_github/CUSUM/output/events/event_00733.csv", path "D:/Analysis/CUSUM_github/CUSUM/output/events/event_00735.csv", path "D:/Analysis/CUSUM_github/CUSUM/output/events/event_00736.csv", path "D:/Analysis/CUSUM_github/CUSUM/output/events/event_00739.csv", path "D:/Analysis/CUSUM_github/CUSUM/output/events/event_00740.csv", path "D:/Analysis/CUSUM_github/CUSUM/output/events/event_00746.csv", path "D:/Analysis/CUSUM_github/CUSUM/output/events/event_00747.csv", path "D:/Analysis/CUSUM_github/CUSUM/output/events/event_00749.csv", path "D:/Analysis/CUSUM_github/CUSUM/output/events/event_00750.csv", path "D:/Analysis/CUSUM_github/CUSUM/output/events/event_00751.csv", path "D:/Analysis/CUSUM_github/CUSUM/output/events/event_00752.csv", path "D:/Analysis/CUSUM_github/CUSUM/output/events/event_00753.csv", path "D:/Analysis/CUSUM_github/CUSUM/output/events/event_00754.csv", path "D:/Analysis/CUSUM_github/CUSUM/output/events/event_00755.csv", path "D:/Analysis/CUSUM_github/CUSUM/output/events/event_00760.csv", path "D:/Analysis/CUSUM_github/CUSUM/output/events/event_00761.csv", path "D:/Analysis/CUSUM_github/CUSUM/output/events/event_00762.csv", path "D:/Analysis/CUSUM_github/CUSUM/output/events/event_00763.csv", path "D:/Analysis/CUSUM_github/CUSUM/output/events/event_00764.csv", path "D:/Analysis/CUSUM_github/CUSUM/output/events/event_00765.csv", path "D:/Analysis/CUSUM_github/CUSUM/output/events/event_00766.csv", path "D:/Analysis/CUSUM_github/CUSUM/output/events/event_00767.csv", path "D:/Analysis/CUSUM_github/CUSUM/output/events/event_00768.csv", path "D:/Analysis/CUSUM_github/CUSUM/output/events/event_00769.csv", path "D:/Analysis/CUSUM_github/CUSUM/output/events/event_00770.csv", path "D:/Analysis/CUSUM_github/CUSUM/output/events/event_00771.csv", path "D:/Analysis/CUSUM_github/CUSUM/output/events/event_00772.csv", path "D:/Analysis/CUSUM_github/CUSUM/output/events/event_00774.csv", path "D:/Analysis/CUSUM_github/CUSUM/output/events/event_00778.csv", path "D:/Analysis/CUSUM_github/CUSUM/output/events/event_00779.csv", path "D:/Analysis/CUSUM_github/CUSUM/output/events/event_00780.csv", path "D:/Analysis/CUSUM_github/CUSUM/output/events/event_00790.csv", path "D:/Analysis/CUSUM_github/CUSUM/output/events/event_00795.csv", path "D:/Analysis/CUSUM_github/CUSUM/output/events/event_00801.csv", path "D:/Analysis/CUSUM_github/CUSUM/output/events/event_00803.csv", path "D:/Analysis/CUSUM_github/CUSUM/output/events/event_00804.csv", path "D:/Analysis/CUSUM_github/CUSUM/output/events/event_00815.csv", path "D:/Analysis/CUSUM_github/CUSUM/output/events/event_00816.csv", path "D:/Analysis/CUSUM_github/CUSUM/output/events/event_00819.csv", path "D:/Analysis/CUSUM_github/CUSUM/output/events/event_00823.csv", path "D:/Analysis/CUSUM_github/CUSUM/output/events/event_00824.csv", path "D:/Analysis/CUSUM_github/CUSUM/output/events/event_00833.csv", path "D:/Analysis/CUSUM_github/CUSUM/output/events/event_00835.csv", path "D:/Analysis/CUSUM_github/CUSUM/output/events/event_00836.csv", path "D:/Analysis/CUSUM_github/CUSUM/output/events/event_00837.csv", path "D:/Analysis/CUSUM_github/CUSUM/output/events/event_00839.csv", path "D:/Analysis/CUSUM_github/CUSUM/output/events/event_00842.csv", path "D:/Analysis/CUSUM_github/CUSUM/output/events/event_00844.csv", path "D:/Analysis/CUSUM_github/CUSUM/output/events/event_00845.csv", path "D:/Analysis/CUSUM_github/CUSUM/output/events/event_00847.csv", path "D:/Analysis/CUSUM_github/CUSUM/output/events/event_00849.csv", path "D:/Analysis/CUSUM_github/CUSUM/output/events/event_00850.csv", path "D:/Analysis/CUSUM_github/CUSUM/output/events/event_00853.csv", path "D:/Analysis/CUSUM_github/CUSUM/output/events/event_00856.csv", path "D:/Analysis/CUSUM_github/CUSUM/output/events/event_00857.csv", path "D:/Analysis/CUSUM_github/CUSUM/output/events/event_00858.csv", path "D:/Analysis/CUSUM_github/CUSUM/output/events/event_00859.csv", path "D:/Analysis/CUSUM_github/CUSUM/output/events/event_00860.csv", path "D:/Analysis/CUSUM_github/CUSUM/output/events/event_00861.csv", path "D:/Analysis/CUSUM_github/CUSUM/output/events/event_00864.csv", path "D:/Analysis/CUSUM_github/CUSUM/output/events/event_00865.csv", path "D:/Analysis/CUSUM_github/CUSUM/output/events/event_00866.csv", path "D:/Analysis/CUSUM_github/CUSUM/output/events/event_00867.csv", path "D:/Analysis/CUSUM_github/CUSUM/output/events/event_00875.csv", path "D:/Analysis/CUSUM_github/CUSUM/output/events/event_00877.csv", path "D:/Analysis/CUSUM_github/CUSUM/output/events/event_00878.csv", path "D:/Analysis/CUSUM_github/CUSUM/output/events/event_00879.csv", path "D:/Analysis/CUSUM_github/CUSUM/output/events/event_00882.csv", path "D:/Analysis/CUSUM_github/CUSUM/output/events/event_00884.csv", path "D:/Analysis/CUSUM_github/CUSUM/output/events/event_00885.csv", path "D:/Analysis/CUSUM_github/CUSUM/output/events/event_00886.csv", path "D:/Analysis/CUSUM_github/CUSUM/output/events/event_00887.csv", path "D:/Analysis/CUSUM_github/CUSUM/output/events/event_00888.csv", path "D:/Analysis/CUSUM_github/CUSUM/output/events/event_00890.csv", path "D:/Analysis/CUSUM_github/CUSUM/output/events/event_00894.csv", path "D:/Analysis/CUSUM_github/CUSUM/output/events/event_00898.csv", path "D:/Analysis/CUSUM_github/CUSUM/output/events/event_00900.csv", path "D:/Analysis/CUSUM_github/CUSUM/output/events/event_00903.csv", path "D:/Analysis/CUSUM_github/CUSUM/output/events/event_00905.csv", path "D:/Analysis/CUSUM_github/CUSUM/output/events/event_00906.csv", path "D:/Analysis/CUSUM_github/CUSUM/output/events/event_00907.csv", path "D:/Analysis/CUSUM_github/CUSUM/output/events/event_00908.csv", path "D:/Analysis/CUSUM_github/CUSUM/output/events/event_00909.csv", path "D:/Analysis/CUSUM_github/CUSUM/output/events/event_00913.csv", path "D:/Analysis/CUSUM_github/CUSUM/output/events/event_00915.csv", path "D:/Analysis/CUSUM_github/CUSUM/output/events/event_00916.csv", path "D:/Analysis/CUSUM_github/CUSUM/output/events/event_00920.csv", path "D:/Analysis/CUSUM_github/CUSUM/output/events/event_00921.csv", path "D:/Analysis/CUSUM_github/CUSUM/output/events/event_00924.csv", path "D:/Analysis/CUSUM_github/CUSUM/output/events/event_00925.csv", path "D:/Analysis/CUSUM_github/CUSUM/output/events/event_00930.csv", path "D:/Analysis/CUSUM_github/CUSUM/output/events/event_00934.csv", path "D:/Analysis/CUSUM_github/CUSUM/output/events/event_00938.csv", path "D:/Analysis/CUSUM_github/CUSUM/output/events/event_00939.csv", path "D:/Analysis/CUSUM_github/CUSUM/output/events/event_00941.csv", path "D:/Analysis/CUSUM_github/CUSUM/output/events/event_00942.csv", path "D:/Analysis/CUSUM_github/CUSUM/output/events/event_00946.csv", path "D:/Analysis/CUSUM_github/CUSUM/output/events/event_00949.csv", path "D:/Analysis/CUSUM_github/CUSUM/output/events/event_00950.csv", path "D:/Analysis/CUSUM_github/CUSUM/output/events/event_00951.csv", path "D:/Analysis/CUSUM_github/CUSUM/output/events/event_00953.csv", path "D:/Analysis/CUSUM_github/CUSUM/output/events/event_00960.csv", path "D:/Analysis/CUSUM_github/CUSUM/output/events/event_00962.csv", path "D:/Analysis/CUSUM_github/CUSUM/output/events/event_00966.csv", path "D:/Analysis/CUSUM_github/CUSUM/output/events/event_00969.csv", path "D:/Analysis/CUSUM_github/CUSUM/output/events/event_00973.csv", path "D:/Analysis/CUSUM_github/CUSUM/output/events/event_00977.csv", path "D:/Analysis/CUSUM_github/CUSUM/output/events/event_00980.csv", path "D:/Analysis/CUSUM_github/CUSUM/output/events/event_00981.csv", path "D:/Analysis/CUSUM_github/CUSUM/output/events/event_00982.csv", path "D:/Analysis/CUSUM_github/CUSUM/output/events/event_00986.csv", path "D:/Analysis/CUSUM_github/CUSUM/output/events/event_00988.csv", path "D:/Analysis/CUSUM_github/CUSUM/output/events/event_00993.csv", path "D:/Analysis/CUSUM_github/CUSUM/output/events/event_00995.csv", path "D:/Analysis/CUSUM_github/CUSUM/output/events/event_00997.csv", path "D:/Analysis/CUSUM_github/CUSUM/output/events/event_00999.csv", path "D:/Analysis/CUSUM_github/CUSUM/output/events/event_01003.csv", path "D:/Analysis/CUSUM_github/CUSUM/output/events/event_01005.csv", path "D:/Analysis/CUSUM_github/CUSUM/output/events/event_01007.csv", path "D:/Analysis/CUSUM_github/CUSUM/output/events/event_01009.csv", path "D:/Analysis/CUSUM_github/CUSUM/output/events/event_01015.csv", path "D:/Analysis/CUSUM_github/CUSUM/output/events/event_01020.csv", path "D:/Analysis/CUSUM_github/CUSUM/output/events/event_01021.csv", path "D:/Analysis/CUSUM_github/CUSUM/output/events/event_01023.csv", path "D:/Analysis/CUSUM_github/CUSUM/output/events/event_01028.csv", path "D:/Analysis/CUSUM_github/CUSUM/output/events/event_01032.csv", path "D:/Analysis/CUSUM_github/CUSUM/output/events/event_01034.csv", path "D:/Analysis/CUSUM_github/CUSUM/output/events/event_01036.csv", path "D:/Analysis/CUSUM_github/CUSUM/output/events/event_01037.csv", path "D:/Analysis/CUSUM_github/CUSUM/output/events/event_01038.csv", path "D:/Analysis/CUSUM_github/CUSUM/output/events/event_01042.csv", path "D:/Analysis/CUSUM_github/CUSUM/output/events/event_01044.csv", path "D:/Analysis/CUSUM_github/CUSUM/output/events/event_01045.csv", path "D:/Analysis/CUSUM_github/CUSUM/output/events/event_01046.csv", path "D:/Analysis/CUSUM_github/CUSUM/output/events/event_01047.csv", path "D:/Analysis/CUSUM_github/CUSUM/output/events/event_01048.csv", path "D:/Analysis/CUSUM_github/CUSUM/output/events/event_01049.csv", path "D:/Analysis/CUSUM_github/CUSUM/output/events/event_01054.csv", path "D:/Analysis/CUSUM_github/CUSUM/output/events/event_01057.csv", path "D:/Analysis/CUSUM_github/CUSUM/output/events/event_01062.csv", path "D:/Analysis/CUSUM_github/CUSUM/output/events/event_01064.csv", path "D:/Analysis/CUSUM_github/CUSUM/output/events/event_01066.csv", path "D:/Analysis/CUSUM_github/CUSUM/output/events/event_01068.csv", path "D:/Analysis/CUSUM_github/CUSUM/output/events/event_01071.csv", path "D:/Analysis/CUSUM_github/CUSUM/output/events/event_01076.csv", path "D:/Analysis/CUSUM_github/CUSUM/output/events/event_01081.csv", path "D:/Analysis/CUSUM_github/CUSUM/output/events/event_01083.csv", path "D:/Analysis/CUSUM_github/CUSUM/output/events/event_01084.csv", path "D:/Analysis/CUSUM_github/CUSUM/output/events/event_01086.csv", path "D:/Analysis/CUSUM_github/CUSUM/output/events/event_01093.csv", path "D:/Analysis/CUSUM_github/CUSUM/output/events/event_01094.csv", path "D:/Analysis/CUSUM_github/CUSUM/output/events/event_01096.csv", path "D:/Analysis/CUSUM_github/CUSUM/output/events/event_01097.csv", path "D:/Analysis/CUSUM_github/CUSUM/output/events/event_01099.csv", path "D:/Analysis/CUSUM_github/CUSUM/output/events/event_01101.csv", path "D:/Analysis/CUSUM_github/CUSUM/output/events/event_01102.csv", path "D:/Analysis/CUSUM_github/CUSUM/output/events/event_01108.csv"]
  out "Total # of events":i32=484
  in  "CUSUM event summary file":path=path "D:/Analysis/CUSUM_github/CUSUM/output/events.csv"
  # "'Page up/down' to \nscan through events"
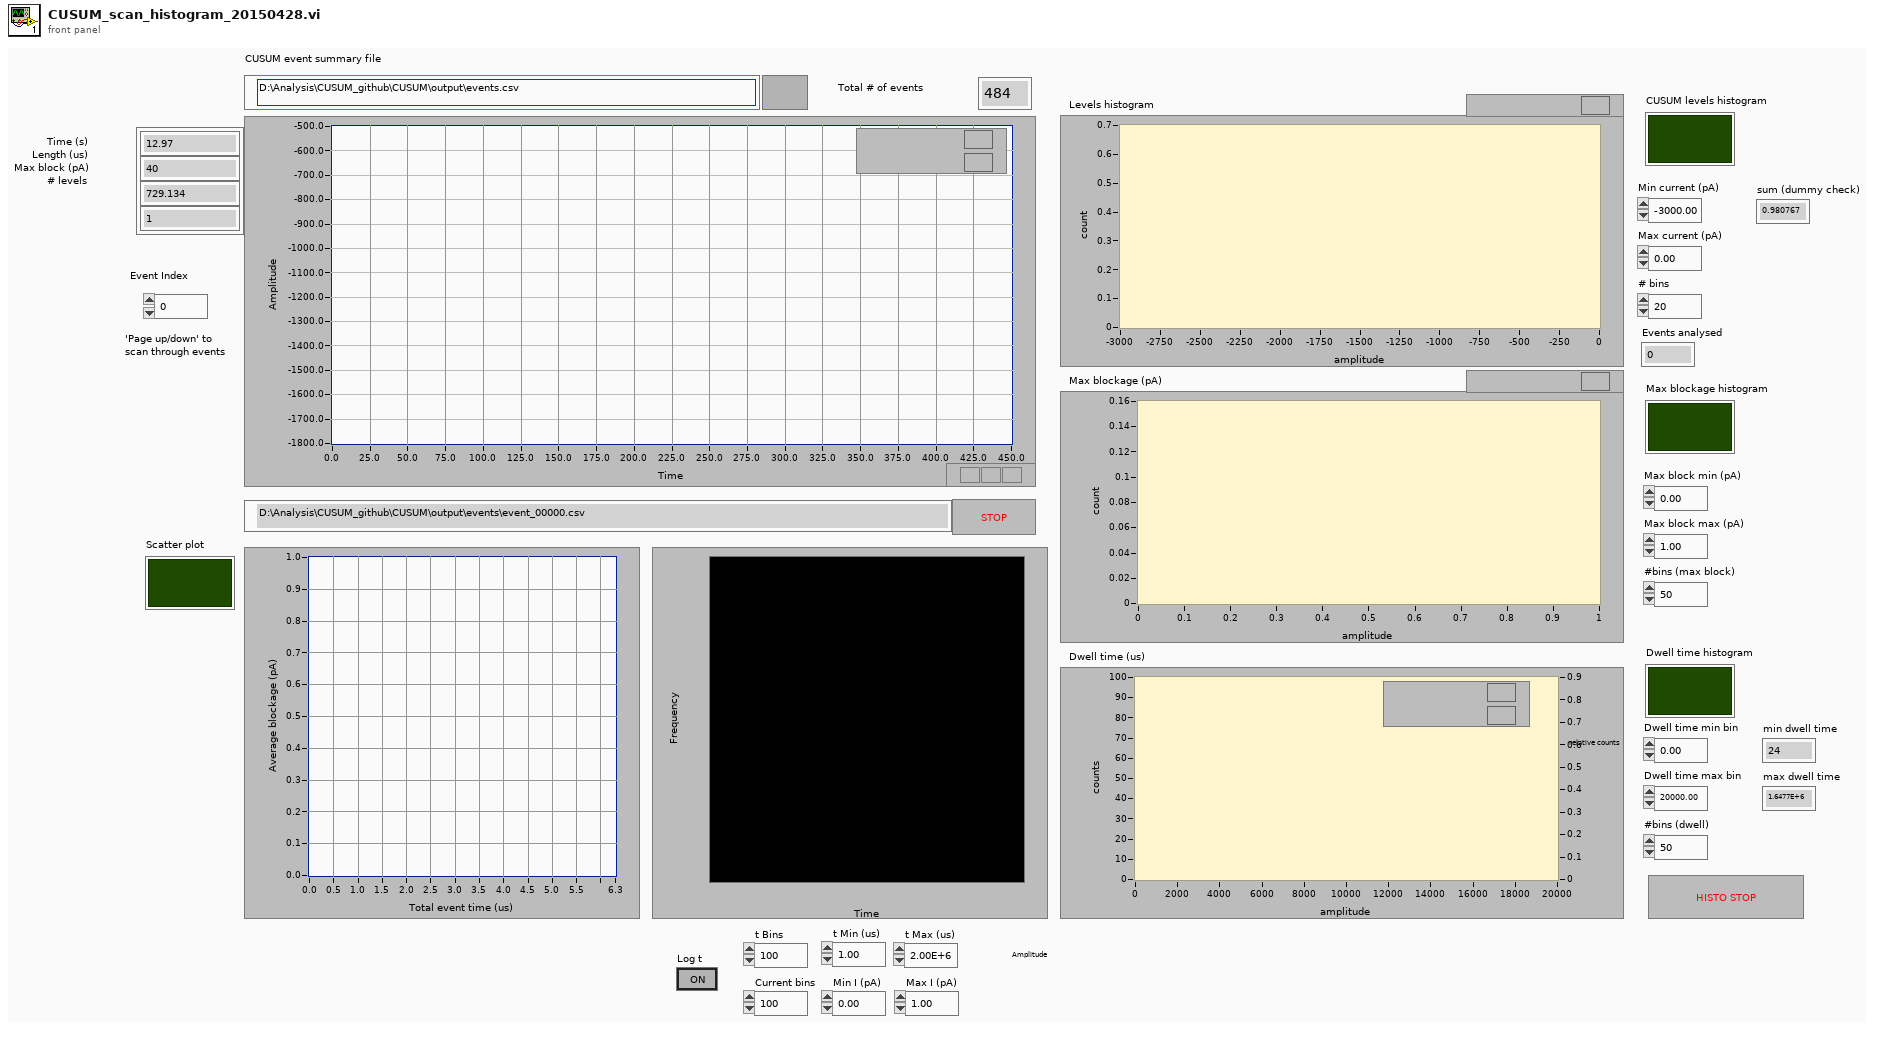
[diagram p1: front panel]
types:
  T1 = cluster{"X Values":dbl[], "Histogram: h(x)":dbl[]}
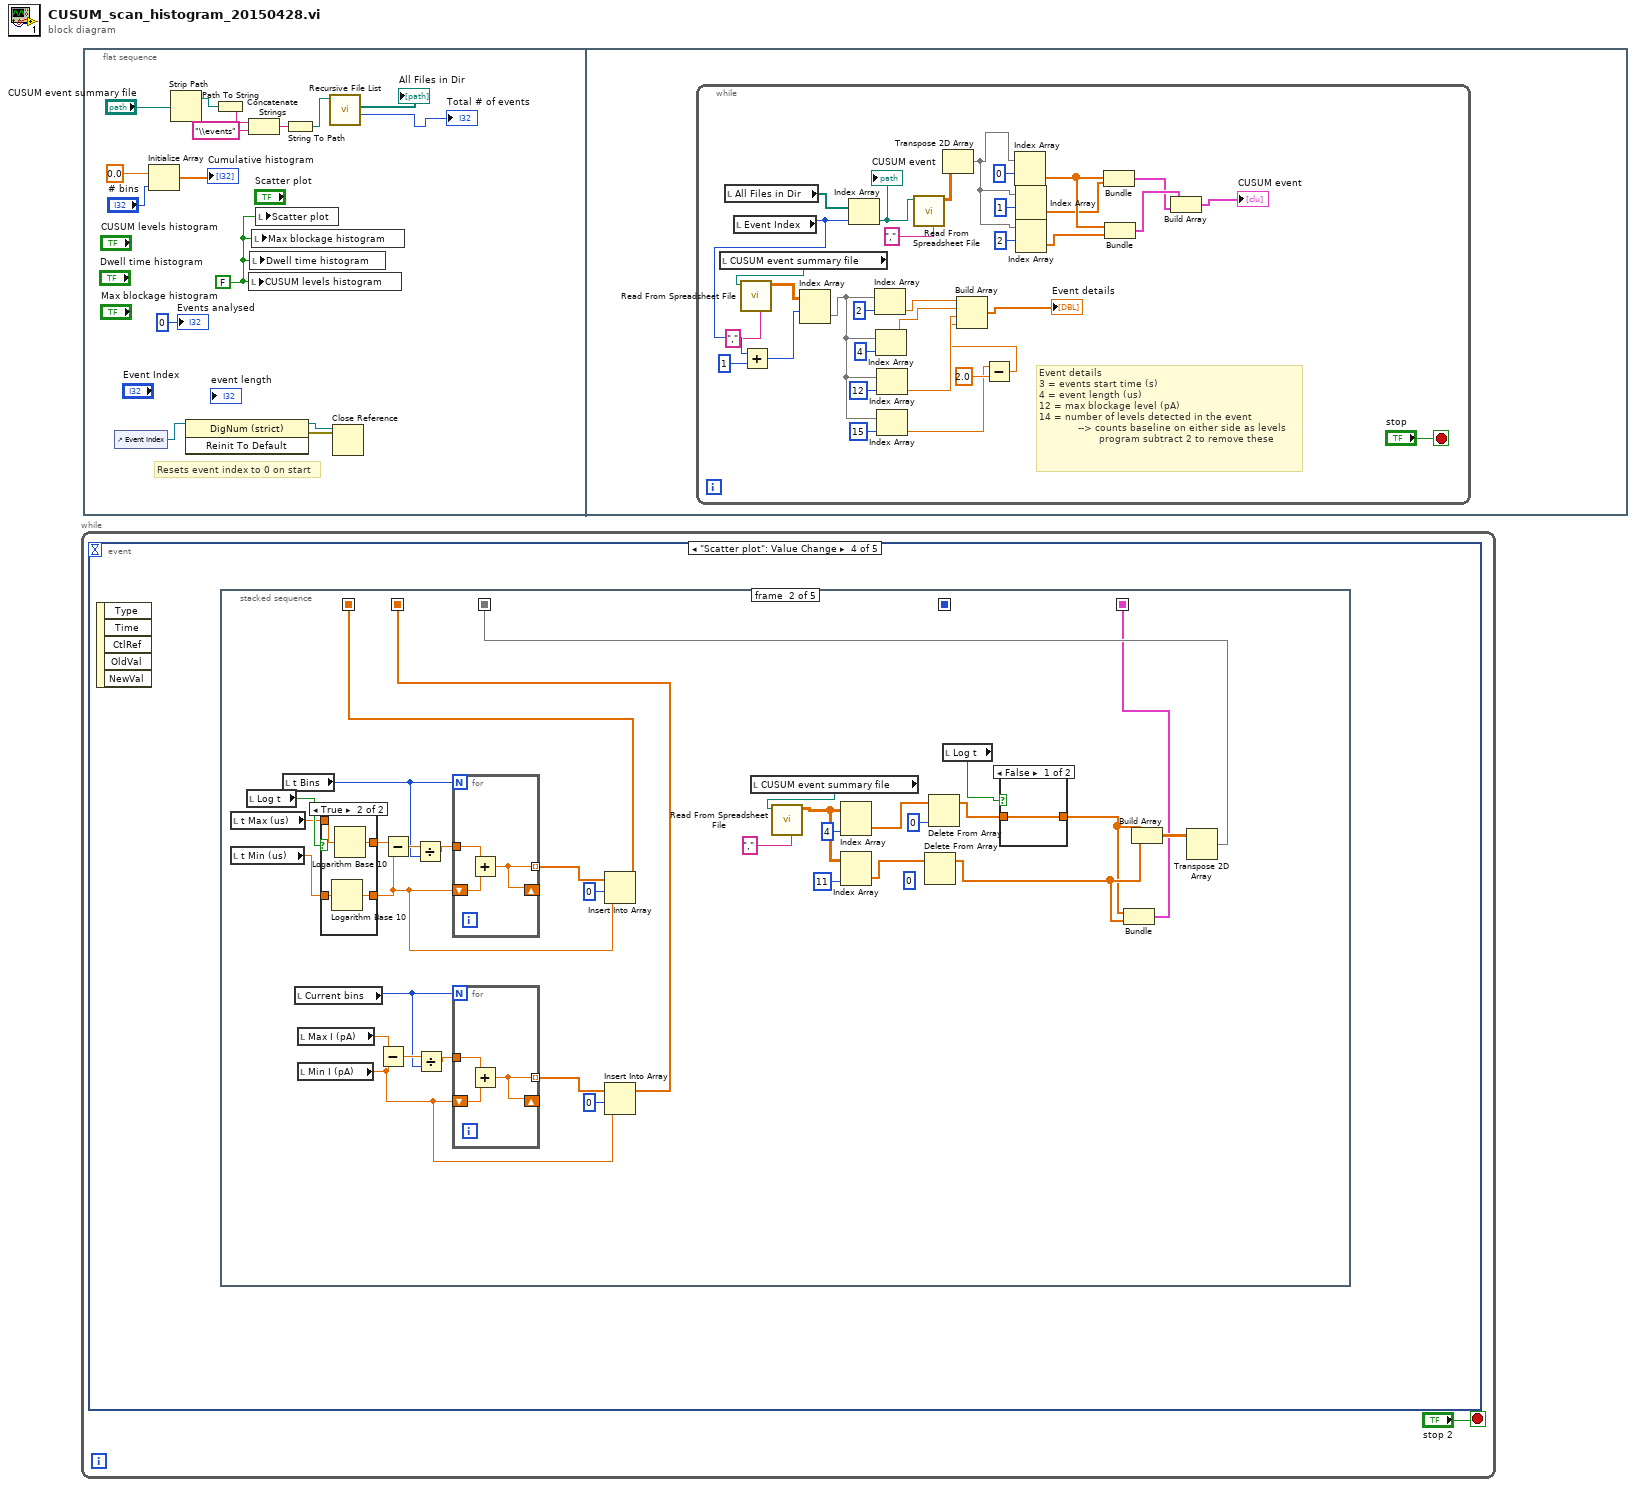
[diagram p0: block diagram]
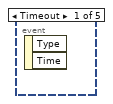
[diagram p2: hidden frame]
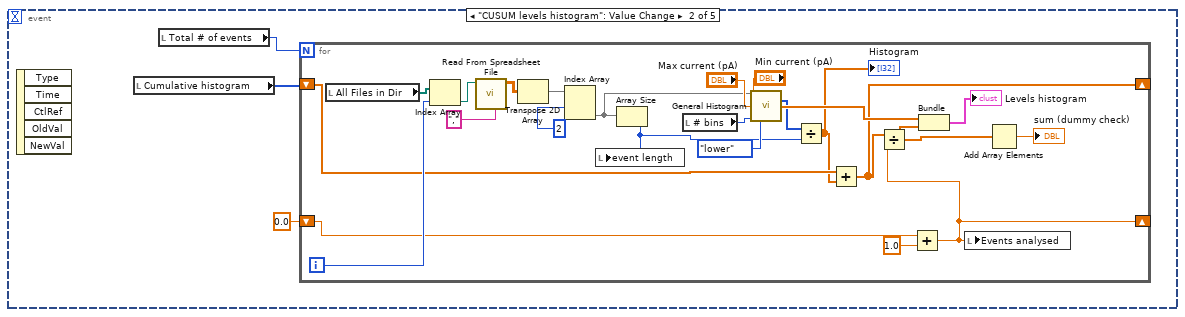
[diagram p3: hidden frame]
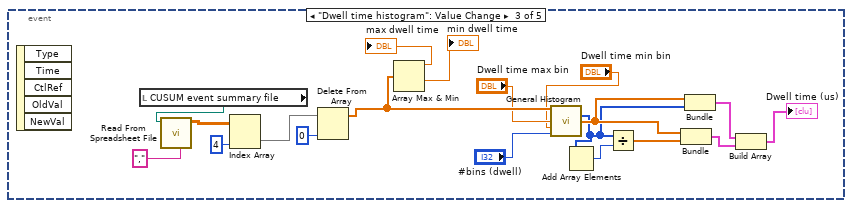
[diagram p4: hidden frame]
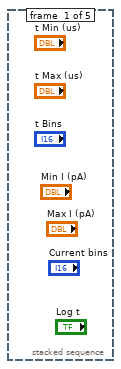
[diagram p5: hidden frame]
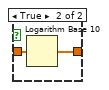
[diagram p6: hidden frame]
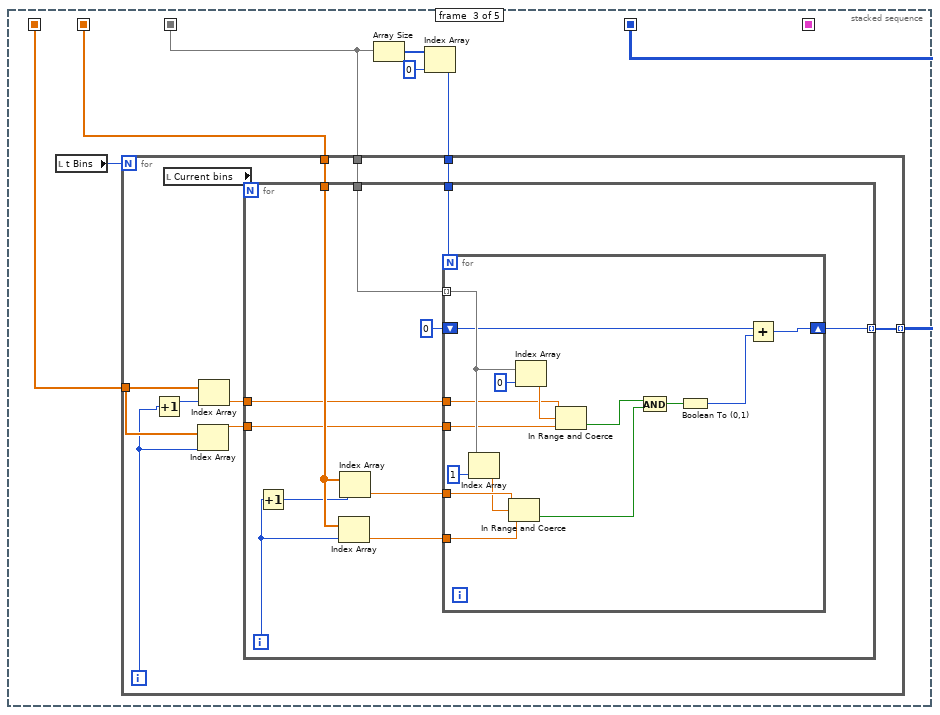
[diagram p8: hidden frame]
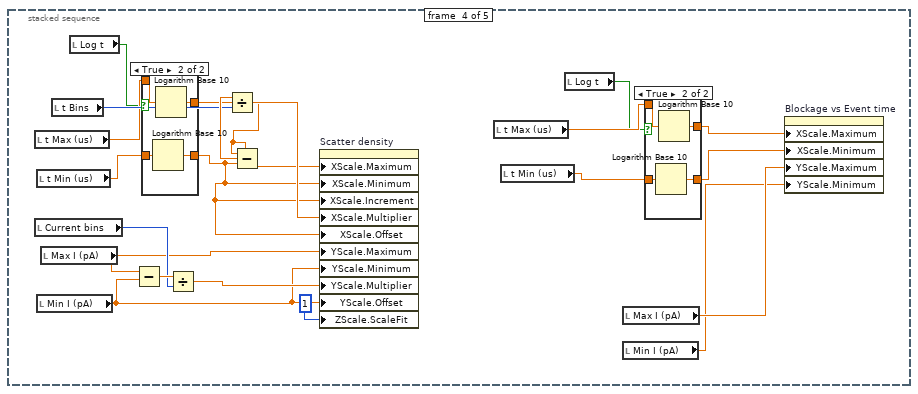
[diagram p9: hidden frame]
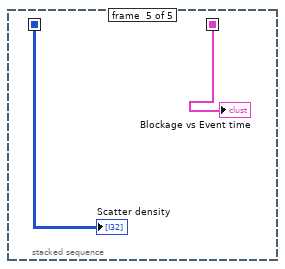
[diagram p12: hidden frame]
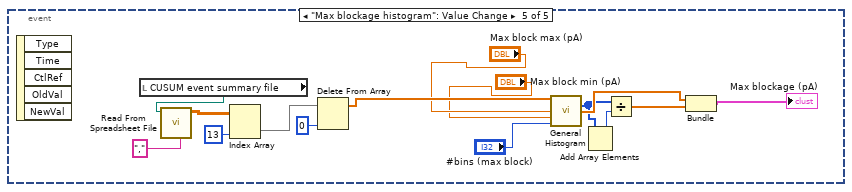
[diagram p13: hidden frame]
diagram:
  n1 = while {
    stop <- "stop 2" stop-if-true
    n2 = event shown="[3] \"Scatter plot\": Value Change" {
      selector: _ -> [_ _ _ _ _]
      dyn-events: _ -> [_ _ _ _ _]
      timeout: _ -> [_ _ _ _ _]
      event Timeout {
        n3 = event-data() -> ()  [unwired: 1 in, 2 out]
      }
      event "CUSUM levels histogram": Value Change {
        n4 = event-data() -> ()  [unwired: 1 in, 5 out]
        n5 = local read "Cumulative histogram"() -> (w3:i32[])
        n6 = local read "Total # of events"() -> (w4:i32)
        n7 = for {
          N: w4 -> [_]
          shift-right: [w10] -> _
          shift-left: w3 -> [w13]
          shift-right: [w6] -> _
          shift-left: 0.0 -> [w8]
          i -> [w28]
          n8 = local read "All Files in Dir"() -> (w27:path[])
          n9 = Index Array(array=w27, index=w28) -> (element=w26:path)
          n10 = call-poly <vilib>:"Read From Spreadsheet File.vi"("delimiter (\\t)"="," ("delimiter (\\t)"), "file path (dialog if empty)"=w26) -> ("all rows"=w21:dbl[][])  [unwired: 5 in, 4 out]
          n11 = Transpose 2D Array(2D array=w21) -> (transposed array=w20:dbl[][])
          n12 = Index Array(array=w20, index (row)=2 ("index")) -> (element=w17:dbl[])  [unwired: 1 in]
          n13 = Array Size(array=w17) -> (size(s)=w15:i32)
          n14 = local write "event length"(w15) -> ()
          n15 = local read "# bins"() -> (w14:i32)
          n16 = call <vilib>:"General Histogram.vi"("X"=w17, "max"="Max current (pA)", "min"="Min current (pA)", "# bins"=w14, "inclusion"=enum32{"lower", "upper"}."lower") -> ("Histogram"=w16:i32[], "Axis"=w19:dbl[])  [unwired: 6 in, 3 out]
          n17 = Divide(x=w16, y=w15) -> (x/y=w11:dbl[])
          "Histogram" <- w11
          n18 = Add(x=w13, y=w11) -> (x+y=w10:dbl[])
          n19 = Add(x=w8, y=1.0) -> (x+y=w6:dbl)
          n20 = Divide(x=w10, y=w6) -> (x/y=w9:dbl[])
          n21 = Bundle("Axis"=w19, w9) -> (→"Levels histogram":cluster{"Axis":dbl[], dbl[]})  [unwired: 1 in]
          n22 = local write "Events analysed"(w6) -> ()
          n23 = Add Array Elements(numeric array=w9) -> (sum=→"sum (dummy check)":dbl)
        }
      }
      event "Dwell time histogram": Value Change {
        n24 = event-data() -> ()  [unwired: 1 in, 5 out]
        n25 = local read "CUSUM event summary file"() -> (w46:path)
        n26 = call-poly <vilib>:"Read From Spreadsheet File.vi"("delimiter (\\t)"="," ("delimiter (\\t)"), "file path (dialog if empty)"=w46) -> ("all rows"=w47:dbl[][])  [unwired: 5 in, 4 out]
        n27 = Index Array(array=w47, index (col)=4 ("disabled index (col)")) -> (element=w44:dbl[])  [unwired: 1 in]
        n28 = Delete From Array(array=w44, index=0) -> (array with subset deleted=w42:dbl[])  [unwired: 1 in, 1 out]
        n29 = Array Max & Min(array=w42) -> (max value=→"max dwell time":dbl, min value=→"min dwell time":dbl)  [unwired: 2 out]
        n30 = call <vilib>:"General Histogram.vi"("X"=w42, "max"="Dwell time max bin", "min"="Dwell time min bin", "# bins"="#bins (dwell)") -> ("Histogram"=w31:i32[], "Axis"=w34:dbl[])  [unwired: 7 in, 3 out]
        n31 = Add Array Elements(numeric array=w31) -> (sum=w30:i32)
        n32 = Divide(x=w31, y=w30) -> (x/y=w38:dbl[])
        n33 = Bundle("Axis"=w34, w38) -> (w33:cluster{"Axis":dbl[], dbl[]})  [unwired: 1 in]
        n34 = Bundle("Axis"=w34, "Histogram"=w31) -> (w32:cluster{"Axis":dbl[], "Histogram":i32[]})  [unwired: 1 in]
        n35 = Build Array(w32, w33) -> (→"Dwell time (us)":cluster{"Axis":dbl[], "Histogram":dbl[]}[])
      }
      event "Scatter plot": Value Change {
        n36 = event-data() -> ()  [unwired: 1 in, 5 out]
        n37 = stacked-sequence {
          seq-local: [_ w78 _ _ _] -> [_ _ w103 _ _]
          seq-local: [_ w72 _ _ _] -> [_ _ w98 _ _]
          seq-local: [_ w74 _ _ _] -> [_ _ w102 _ _]
          seq-local: [_ _ w97 _ _] -> [_ _ _ _ w175]
          seq-local: [_ w57 _ _ _] -> [_ _ _ _ w174]
          frame #0 {
          }
          frame #1 {
            (unwired) 0 ("index")
            n38 = local read "t Max (us)"() -> (w55:dbl)
            n39 = local read "t Min (us)"() -> (w53:dbl)
            n40 = local read "Log t"() -> (w56:bool)
            n41 = local read "t Bins"() -> (w70:i16)
            n42 = local read "Current bins"() -> (w66:i16)
            n43 = local read "Max I (pA)"() -> (w81:dbl)
            n44 = local read "Min I (pA)"() -> (w75:dbl)
            n45 = case shown="True" w56 {
              tunnel: w55 -> [w86 w90]
              tunnel: [w86 w89] -> w54
              tunnel: w53 -> [w85 w88]
              tunnel: [w85 w87] -> w52
              frame False {
              }
              frame True {
                n46 = Logarithm Base 10(1:w88) -> (0:w87:dbl)
                n47 = Logarithm Base 10(1:w90) -> (0:w89:dbl)
              }
            }
            n48 = Subtract(x=w81, y=w75) -> (x-y=w68:dbl)
            n49 = Subtract(x=w54, y=w52) -> (x-y=w71:dbl)
            n50 = Divide(x=w71, y=w70) -> (x/y=w69:dbl)
            n51 = Divide(x=w68, y=w66) -> (x/y=w67:dbl)
            n52 = for {
              N: w70 -> [_]
              tunnel: w69 -> [w96]
              shift-right: [w94] -> _
              shift-left: w52 -> [w95]
              tunnel: [w94] -> w80 mode=indexing
              n53 = Add(x=w96, y=w95) -> (x+y=w94:dbl)
            }
            n54 = for {
              N: w66 -> [_]
              tunnel: w67 -> [w93]
              shift-right: [w91] -> _
              shift-left: w75 -> [w92]
              tunnel: [w91] -> w76 mode=indexing
              n55 = Add(x=w93, y=w92) -> (x+y=w91:dbl)
            }
            n56 = Insert Into Array(array=w80, index=0, new element=w52) -> (w78:dbl[])
            n57 = Insert Into Array(array=w76, index=0, new element=w75) -> (w74:dbl[])
            n58 = local read "CUSUM event summary file"() -> (w59:path)
            n59 = call-poly <vilib>:"Read From Spreadsheet File.vi"("delimiter (\\t)"="," ("delimiter (\\t)"), "file path (dialog if empty)"=w59) -> ("all rows"=w64:dbl[][])  [unwired: 5 in, 4 out]
            n60 = Index Array(array=w64, index (col)=4 ("disabled index (col)")) -> (element=w61:dbl[])  [unwired: 1 in]
            n61 = Index Array(array=w64, index (col)=11) -> (element=w65:dbl[])  [unwired: 1 in]
            n62 = Delete From Array(array=w65) -> (array with subset deleted=w58:dbl[])  [unwired: 2 in, 1 out]
            n63 = Delete From Array(array=w61, index=0) -> (array with subset deleted=w51:dbl[])  [unwired: 1 in, 1 out]
            n64 = local read "Log t"() -> (w49:bool)
            n65 = case shown="False" w49 {
              tunnel: w51 -> [w82 w84]
              tunnel: [w82 w83] -> w50
              frame False {
              }
              frame True {
                n66 = Logarithm Base 10(1:w84) -> (0:w83:dbl[])
              }
            }
            n67 = Bundle("all rows"=w50, "all rows"=w58) -> (w57:cluster{"all rows":dbl[], "all rows":dbl[]})  [unwired: 1 in]
            n68 = Build Array(w50, w58) -> (w73:dbl[][])
            n69 = Transpose 2D Array(2D array=w73) -> (transposed array=w72:dbl[][])
          }
          frame #2 {
            n70 = local read "t Bins"() -> (w104:i16)
            n71 = Array Size(array=w98) -> (size(s)=w101:i32[])
            n72 = Index Array(array=w101, index=0) -> (element=w99:i32)
            n73 = for {
              N: w104 -> [_]
              tunnel: w103 -> [w114]
              tunnel: w102 -> [w112]
              tunnel: w99 -> [w111]
              tunnel: w98 -> [w110]
              tunnel: [w107] -> w97 mode=indexing
              i -> [w105]
              n74 = Increment(x=w105) -> (x+1=w106:i32)
              n75 = local read "Current bins"() -> (w113:i16)
              n76 = Index Array(array=w114, index=w105) -> (element=w108:dbl)
              n77 = Index Array(array=w114, index=w106) -> (element=w109:dbl)
              n78 = for {
                N: w113 -> [_]
                tunnel: w112 -> [w125]
                tunnel: w111 -> [w124]
                tunnel: w110 -> [w123]
                tunnel: w109 -> [w119]
                tunnel: w108 -> [w118]
                tunnel: [w117] -> w107 mode=indexing
                i -> [w116]
                n79 = Increment(x=w116) -> (x+1=w115:i32)
                n80 = Index Array(array=w125, index=w116) -> (element=w120:dbl)
                n81 = Index Array(array=w125, index=w115) -> (element=w121:dbl)
                n82 = for {
                  N: w124 -> [_]
                  tunnel: w123 -> [w134] mode=indexing
                  shift-right: [w126] -> w117
                  shift-left: 0 -> [w127]
                  tunnel: w121 -> [w140]
                  tunnel: w120 -> [w139]
                  tunnel: w119 -> [w133]
                  tunnel: w118 -> [w132]
                  n83 = Index Array(array=w134, index=1) -> (element=w137:dbl)
                  n84 = In Range and Coerce(upper limit=w140, x=w137, lower limit=w139) -> (In Range?=w130:bool)  [unwired: 1 out]
                  n85 = Index Array(array=w134, index=0) -> (element=w136:dbl)
                  n86 = In Range and Coerce(upper limit=w133, x=w136, lower limit=w132) -> (In Range?=w131:bool)  [unwired: 1 out]
                  n87 = And(x=w131, y=w130) -> (x .and. y?=w129:bool)
                  n88 = Boolean To (0,1)(Boolean=w129) -> (0, 1=w128:i16)
                  n89 = Add(x=w127, y=w128) -> (x+y=w126:i32)
                }
              }
            }
          }
          frame #3 {
            n90 = local read "t Max (us)"() -> (w150:dbl)
            n91 = local read "Current bins"() -> (w159:i16)
            n92 = local read "t Min (us)"() -> (w149:dbl)
            n93 = local read "Min I (pA)"() -> (w153:dbl)
            n94 = local read "Max I (pA)"() -> (w154:dbl)
            n95 = local read "t Bins"() -> (w156:i16)
            n96 = local read "Log t"() -> (w146:bool)
            n97 = Subtract(x=w154, y=w153) -> (x-y=w160:dbl)
            n98 = case shown="True" w146 {
              tunnel: w150 -> [w169 w173]
              tunnel: [w169 w172] -> w147
              tunnel: w149 -> [w168 w171]
              tunnel: [w168 w170] -> w148
              frame False {
              }
              frame True {
                n99 = Logarithm Base 10(1:w171) -> (0:w170:dbl)
                n100 = Logarithm Base 10(1:w173) -> (0:w172:dbl)
              }
            }
            n101 = Divide(x=w160, y=w159) -> (x/y=w158:dbl)
            n102 = Subtract(x=w147, y=w148) -> (x-y=w157:dbl)
            n103 = Divide(x=w157, y=w156) -> (x/y=w155:dbl)
            n104 = property on="Scatter density" class="IntGraph (strict)"("XScale.Maximum"=w147, "XScale.Minimum"=w148, "XScale.Increment"=w148, "XScale.Multiplier"=w155, "XScale.Offset"=w148, "YScale.Maximum"=w154, "YScale.Minimum"=w153, "YScale.Multiplier"=w158, "YScale.Offset"=w153, "ZScale.ScaleFit"=u8 1 ("Z Scale.Scale Fit")) -> ()  [unwired: 2 in, 2 out]
            n105 = local read "t Max (us)"() -> (w145:dbl)
            n106 = local read "t Min (us)"() -> (w143:dbl)
            n107 = local read "Log t"() -> (w141:bool)
            n108 = local read "Max I (pA)"() -> (w152:dbl)
            n109 = local read "Min I (pA)"() -> (w151:dbl)
            n110 = case shown="True" w141 {
              tunnel: w145 -> [w163 w167]
              tunnel: [w163 w166] -> w144
              tunnel: w143 -> [w162 w165]
              tunnel: [w162 w164] -> w142
              frame False {
              }
              frame True {
                n111 = Logarithm Base 10(1:w165) -> (0:w164:dbl)
                n112 = Logarithm Base 10(1:w167) -> (0:w166:dbl)
              }
            }
            n113 = property on="Blockage vs Event time" class="XYGraph (strict)"("XScale.Maximum"=w144, "XScale.Minimum"=w142, "YScale.Maximum"=w152, "YScale.Minimum"=w151) -> ()  [unwired: 2 in, 2 out]
          }
          frame #4 {
            "Scatter density" <- w175
            "Blockage vs Event time" <- w174
          }
        }
      }
      event "Max blockage histogram": Value Change {
        n114 = event-data() -> ()  [unwired: 1 in, 5 out]
        n115 = local read "CUSUM event summary file"() -> (w189:path)
        n116 = call-poly <vilib>:"Read From Spreadsheet File.vi"("delimiter (\\t)"="," ("delimiter (\\t)"), "file path (dialog if empty)"=w189) -> ("all rows"=w190:dbl[][])  [unwired: 5 in, 4 out]
        n117 = Index Array(array=w190, index (col)=13 ("disabled index (col)")) -> (element=w187:dbl[])  [unwired: 1 in]
        n118 = Delete From Array(array=w187, index=0) -> (array with subset deleted=w185:dbl[])  [unwired: 1 in, 1 out]
        n119 = call <vilib>:"General Histogram.vi"("X"=w185, "max"="Max block max (pA)", "min"="Max block min (pA)", "# bins"="#bins (max block)") -> ("Histogram"=w177:i32[], "Axis"=w181:dbl[])  [unwired: 7 in, 3 out]
        n120 = Add Array Elements(numeric array=w177) -> (sum=w178:i32)
        n121 = Divide(x=w177, y=w178) -> (x/y=w182:dbl[])
        n122 = Bundle("Axis"=w181, w182) -> (→"Max blockage (pA)":cluster{"Axis":dbl[], dbl[]})  [unwired: 1 in]
      }
    }
  }
  n123 = flat-sequence {
    frame #0 {
      w197 = FALSE ("Accumulate histogram")
      # "Resets event index to 0 on start"
      n124 = control-ref of="Event Index"() -> (w205:refnum<vi>)
      n125 = Initialize Array(0.0 ("element"), "# bins") -> (→"Cumulative histogram":dbl[])
      n126 = Strip Path(path="CUSUM event summary file") -> (stripped path=w196:path)  [unwired: 1 out]
      n127 = invoke class="DigNum (strict)" method="Reinit To Default"(reference=w205) -> (reference out=w204:refnum<vi>, error out=w203:errorcluster)  [unwired: 2 in, 1 out]
      n128 = Path To String(path=w196) -> (string=w195:string)
      n129 = Concatenate Strings(w195, "\\events" ("string")) -> (w193:string)
      n130 = local write "CUSUM levels histogram"(w197) -> ()
      n131 = local write "Dwell time histogram"(w197) -> ()
      n132 = local write "Max blockage histogram"(w197) -> ()
      n133 = local write "Scatter plot"(w197) -> ()
      n134 = String To Path(string=w193) -> (path=w192:path)
      n135 = call <vilib>:"Recursive File List.vi"("Folder Path"=w192) -> ("Number of Files"=→"Total # of events":i32, "All Files in Dir"=→"All Files in Dir":path[])  [unwired: 6 in, 3 out]
      n136 = Close Reference(reference=w204, error in (no error)=w203) -> ()  [unwired: 1 out]
      "Events analysed" <- 0
    }
    frame #1 {
      n137 = while {
        stop <- "stop" stop-if-true
        # "Event details\n3 = events start time (s)\n4 = event length (us)\n12 = max blockage level (pA)\n14 = number of levels detected in the event\n             --> counts baseline on either side as levels\n                    program subtract 2 to remove these"
        n138 = local read "CUSUM event summary file"() -> (w226:path)
        n139 = local read "All Files in Dir"() -> (w239:path[])
        n140 = local read "Event Index"() -> (w217:i32)
        n141 = call-poly <vilib>:"Read From Spreadsheet File.vi"("delimiter (\\t)"="," ("delimiter (\\t)"), "file path (dialog if empty)"=w226) -> ("all rows"=w225:dbl[][])  [unwired: 5 in, 4 out]
        n142 = Add(x=w217, y=1) -> (x+y=w218:i32)
        n143 = Index Array(array=w225, index (row)=w218) -> (element=w215:dbl[])  [unwired: 1 in]
        n144 = Index Array(array=w239, index=w217) -> (element=w238:path)
        "CUSUM event" <- w238
        n145 = Index Array(array=w215, index=2) -> (element=w224:dbl)
        n146 = Index Array(array=w215, index=4) -> (element=w223:dbl)
        n147 = Index Array(array=w215, index=12) -> (element=w222:dbl)
        n148 = Index Array(array=w215, index=15) -> (element=w212:dbl)
        n149 = call-poly <vilib>:"Read From Spreadsheet File.vi"("delimiter (\\t)"="," ("delimiter (\\t)"), "file path (dialog if empty)"=w238) -> ("all rows"=w230:dbl[][])  [unwired: 5 in, 4 out]
        n150 = Transpose 2D Array(2D array=w230) -> (transposed array=w229:dbl[][])
        n151 = Subtract(x=w212, y=2.0) -> (x-y=w211:dbl)
        n152 = Build Array(w224, w223, w222, w211) -> (→"Event details":dbl[])
        n153 = Index Array(array=w229, index (row)=0 ("index")) -> (element=w234:dbl[])  [unwired: 1 in]
        n154 = Index Array(array=w229, index (row)=1 ("index")) -> (element=w233:dbl[])  [unwired: 1 in]
        n155 = Index Array(array=w229, index (row)=2 ("index")) -> (element=w232:dbl[])  [unwired: 1 in]
        n156 = Bundle(w234, w233) -> (w227:cluster{dbl[], dbl[]})  [unwired: 1 in]
        n157 = Bundle(w234, w232) -> (w228:cluster{dbl[], dbl[]})  [unwired: 1 in]
        n158 = Build Array(w228, w227) -> (→"CUSUM event":cluster{dbl[], dbl[]}[])
      }
    }
  }
